vi "Autonomous Independent.vi"() -> ()   [LabVIEW 2011]
doc: "This VI is called when autonomous begins, and will automatically be terminated when autonomous ends. You can carry out timed or sensor driven robot movement independently without needing to return to the caller."
uses:
  <vilib>/Rock Robotics/WPI/Relay/WPI_RelayValue.ctl
  Robot Global Data.vi
  <vilib>/addons/control/pid/pid.llb/PID (DBL).vi
  <vilib>/addons/control/pid/NI_PID_pid.lvlib
  <vilib>/Analysis/NI_AALBase.lvlib
panel:
  out "RPM Control 3":dbl
  out "Target Distance 3":dbl
  out "Turret Stable? 4":bool
  out "State 4":i32
  out "Numeric 4":i32
  in  "Pulse Width (sec) 4":dbl(knob)=0.5086712930755795 scale=0.0..4.0
  out "In Range? 4":bool
  out "RPM Control 2":dbl
  out "Target Distance 2":dbl
  out "Turret Stable? 3":bool
  out "State 3":i32
  out "Numeric 3":i32
  in  "Pulse Width (sec) 3":dbl(knob)=0.5086712930755795 scale=0.0..4.0
  out "In Range? 3":bool
  out "Report":i32
  out "A2: F2":i32
  out "A2: S2":i32
  out "A2: P2":i32
  out "A2: F1":i32
  out "A2: S1":i32
  out "Prime 1":i32
  out "Edge 1":bool
  out "Count 1":bool
  out "Edge 2":bool
  out "count 2":bool
  out "Fire 1":i32
  out "Shooter Stab 1":i32
  out "Fire":i32
  out "Shooter Stable":i32
  out "RPM Control":dbl
  out "Target Distance":dbl
  out "Shooter RPM Response 2":dbl
  out "Waveform Chart 2":cluster{"Shooter RPM Response":dbl, i16}(graph) caption="Waveform Chart"
  out "Turret Stable? 2":bool
  out "State 2":i32
  out "Numeric 2":i32
  in  "Pulse Width (sec) 2":dbl(knob)=0.5086712930755795 scale=0.0..4.0
  out "In Range? 2":bool
  out "In Range?":bool
  in  "Pulse Width (sec)":dbl(knob)=0.5086712930755795 scale=0.0..4.0
  out "Numeric":i32
  out "Turret Stable?":bool
  out "State":i32
  out "Shooter RPM Response":dbl
  in  "Intake Delay (sec)":dbl(knob)=0.15160369527651382 scale=0.0..1.0
  in  "Auto Target Tol (deg)":dbl=1.0
  out "Auton Mode":u32
  in  "Bridge Ball Timeout (sec) 4":dbl=14.5
  out "x-y 61":dbl
  out "x-y 60":dbl
  in  "Prop 4":dbl(knob)=0.059181315414781936 scale=0.0..0.1
  in  "Int 4":dbl(knob) scale=0.0..0.2
  in  "Deriv 4":dbl(knob)=0.030506642412339725 scale=0.0..0.1
  out "RPM Control Response 4":cluster{"setpoint":dbl, "Angle":dbl}(graph)
  out "PID Output 4":dbl(graph)
  out "x-y 56":dbl
  out "x-y 43":dbl
  out "x-y 42":dbl
  in  "Ball 1 Timeout (sec) 5":dbl=6.0
  in  "Prop 2":dbl(knob)=0.059181315414781936 scale=0.0..0.1
  in  "Int 2":dbl(knob) scale=0.0..0.2
  in  "Deriv 2":dbl(knob)=0.030506642412339725 scale=0.0..0.1
  out "RPM Control Response 2":cluster{"setpoint":dbl, "Angle":dbl}(graph)
  out "PID Output 2":dbl(graph)
  out "x-y 34":dbl
  out "x-y 32":dbl
  out "x-y 31":dbl
  in  "Ball 2 Timeout (sec) 4":dbl=8.0
  out "x-y 30":dbl
  out "x-y 29":dbl
  out "x-y 28":dbl
  in  "Ball 1 Timeout (sec) 4":dbl=6.0
  out "x-y 27":dbl
  out "x-y 26":dbl
  in  "Ball 2 Timeout (sec) 3":dbl=12.0
  out "Shooter Ready? 4":bool
  out "x-y 25":dbl
  out "x-y 24":dbl
  out "x-y 23":dbl
  in  "Ball 1 Timeout (sec) 3":dbl=7.0
  out "x-y 22":dbl
  out "x-y 21":dbl
  out "x-y 20":dbl
  in  "Ball 2 Timeout (sec) 2":dbl=12.0
  out "x-y 19":dbl
  out "x-y 18":dbl
  out "x-y 17":dbl
  in  "Ball 1 Timeout (sec) 2":dbl=7.0
  out "x-y 16":dbl
  out "x-y 15":dbl
  in  "Bridge Timeout (sec)":dbl=10.0
  out "x-y 14":dbl
  in  "Bridge Wait Time":dbl=3.0
  out "x-y 7":dbl
  out "x-y 6":dbl
  out "x-y 5":dbl
  out "x-y 4":dbl
  out "x-y 3":dbl
  out "x-y 2":dbl
  out "x-y":dbl
  in  "Ball 1 Timeout (sec)":dbl=6.0
  in  "Ball 2 Timeout (sec)":dbl=8.0
  out "PID Output":dbl(graph)
  in  "Deriv":dbl(knob)=0.030506642412339725 scale=0.0..0.1
  in  "Int":dbl(knob) scale=0.0..0.2
  in  "Prop":dbl(knob)=0.059181315414781936 scale=0.0..0.1
  out "RPM Control Response":cluster{"setpoint":dbl, "Angle":dbl}(graph)
  in  "Drive Brake 'Speed'":dbl=-0.25
  in  "Bridge Actuator Up Time":dbl=0.7
  in  "Bridge Shooter RPM":dbl(knob)=2375.3275564878513 scale=0.0..3000.0
  in  "Bridge Actuator Down Time":dbl=0.7
  in  "Drive Speed":dbl(knob)=0.7003240287631072 scale=0.0..1.0
  in  "Drive Distance (in)":dbl=52.0
  in  "Key Shooter RPM":dbl(knob)=2129.320851431791 scale=0.0..3000.0
  # "0.00228834"
  # "5.2917"
  # "5.86597"
  # "6.97894"
  # "8.73895"
  # "9.44921"
  # "11.5852"
  # "Tol = 25 RPM"
  # "0.00236416"
  # "5.12686"
  # "5.65754"
  # "6.9858"
  # "9.2698"
  # "9.95681"
  # "12.0508"
  # "Fire Ball 1"
  # "Shooter Stable?"
  # "Drive to Bridge"
  # "Wait for Intake"
  # "Shooter at RPM"
  # "Re-Prime for Ball 2"
  # "Fire Ball 2"
  # "Push Bridge"
  # "0.00585747"
  # "3.96963"
  # "4.19854"
  # "4.7273"
  # "6.06736"
  # "6.50122"
  # "7.63292"
  # "8.43019"
  # "14.7075"
  # "0.0028162"
  # "3.90909"
  # "4.35412"
  # "5.11691"
  # "7.55852"
  # "8.06268"
  # "9.35977"
  # "10.1718"
  # "14.7173"
  # "0.0742593"
  # "4.51218"
  # "5.00045"
  # "5.66034"
  # "7.27621"
  # "7.7194"
  # "9.01324"
  # "0"
  # "0"
  # "7.69482"
  # "12.2315"
  # "12.799"
  # "0.00151539"
  # "7.25307"
  # "8.87523"
  # "14.7224"
  # "Tol = 15 RPM"
  # "11.2711"
  # "11.7239"
  # "8.43608"
  # "6.5389"
  # "7.09492"
  # "13.7465"
  # "0.00176096"
  # "Was 0.25 at St.Louis"
  # "Cheas Match 1 was 48\""
  # "48 Inch from curve of Key to Bridge"
  # "Fairgrounds was 2415"
  # "Cheas Practice was 2325"
  # "Cheas Start was 2375"
  # "At RPM"
  # "Fire B1"
  # "Prime B2"
  # "At RPM"
  # "Fire B2"
  # "Auton #2"
  # "0.12688"
  # "10.6952"
  # "11.3261"
  # "12.7335"
  # "13.8453"
  # "14.5186"
types:
  T1 = typedef "WPI_EncoderDevRef.ctl" = cluster{"DevStatus":errorcluster, "EncoderIndex":T2, "CounterIndex":T3, "DistancePerCount":dbl, "Decoding Type":T4}
  T2 = typedef "FPGA_EncoderIdx.ctl" = enum8{"Enc 0", "Enc 1", "Enc 2", "Enc 3", "Invalid"}
  T3 = typedef "FPGA_CounterCtrSystemIndex.ctl" = enum8{"Ctr 0", "Ctr 1", "Ctr 2", "Ctr 3", "Ctr 4", "Ctr 5", "Ctr 6", "Ctr 7", "Invalid"}
  T4 = typedef "WPI_EncoderType.ctl" = enum16{"1x", "2x", "4x"}
  T5 = typedef "WPI_GyroDevRef.ctl" = cluster{"DevStatus":errorcluster, "Analog Module":T6, "Analog Channel":T7, "Offset":dbl, "Gain (VoltsPerDegree/Second)":dbl}
  T6 = typedef "FPGA_TypedefAnalogModule.ctl" = enum16{"Analog Module 1", "Analog Module 2"}
  T7 = typedef "FPGA_AIChannel.ctl" = enum8{"AI 1", "AI 2", "AI 3", "AI 4", "AI 5", "AI 6", "AI 7", "AI 8", "Invalid"}
  T8 = typedef "WPI_DigitalInputDevRef.ctl" = cluster{"DevStatus":errorcluster, "DIO Channel":T9, "Digital Module":T10}
  T9 = typedef "FPGA_DIOChannel.ctl" = enum8{"DIO 1", "DIO 2", "DIO 3", "DIO 4", "DIO 5", "DIO 6", "DIO 7", "DIO 8", "DIO 9", "DIO 10", "DIO 11", "DIO 12", "DIO 13", "DIO 14", "Invalid"}
  T10 = typedef "FPGA_TypedefDigitalModule.ctl" = enum16{"Digital Module 1", "Digital Module 2"}
  T11 = typedef "WPI_RelayDevRef.ctl" = cluster{"DevStatus":errorcluster, "Relay Channel":T12, "Digital Module":T10, "Relay Direction":T13}
  T12 = typedef "FPGA_DIORelayChannel.ctl" = enum8{"Relay 1", "Relay 2", "Relay 3", "Relay 4", "Relay 5", "Relay 6", "Relay 7", "Relay 8", "Invalid"}
  T13 = typedef "WPI_RelayDirection.ctl" = enum16{"Both directions", "Forward only", "Reverse only"}
  T14 = typedef "WPI_RelayValue.ctl" = enum16{"Off", "On", "Forward", "Reverse"}
  T15 = cluster{"Target Distance":dbl, "Target Distance":dbl, "Target Distance":dbl, "Target Distance":dbl, "Target Distance":dbl}
  T16 = cluster{"Prop 2":dbl, "Int 2":dbl, "Deriv 2":dbl}
  T17 = cluster{"Prop 4":dbl, "Int 4":dbl, "Deriv 4":dbl}
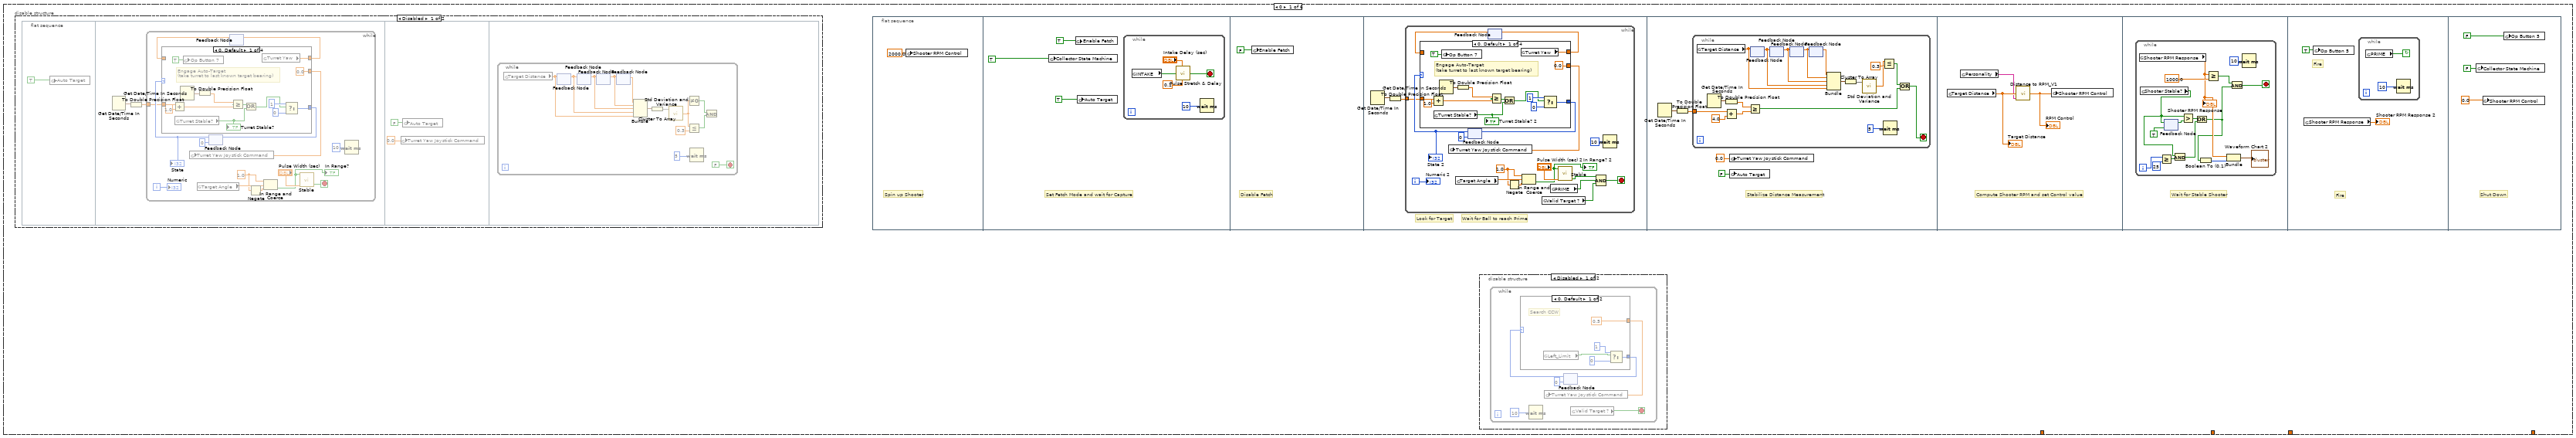
[diagram p2: hidden frame]
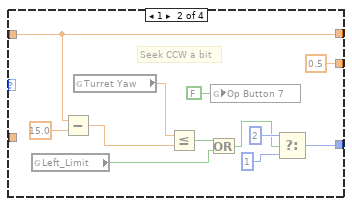
[diagram p3: hidden frame]
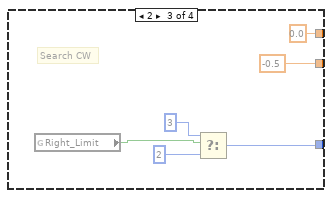
[diagram p4: hidden frame]
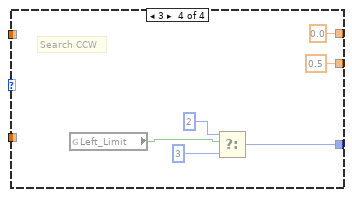
[diagram p5: hidden frame]
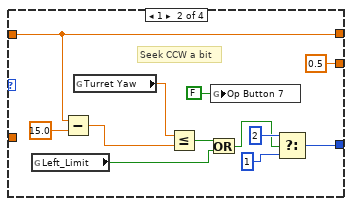
[diagram p7: hidden frame]
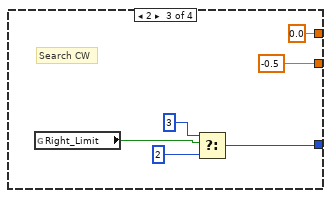
[diagram p8: hidden frame]
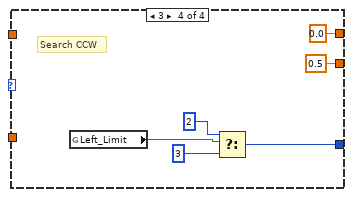
[diagram p9: hidden frame]
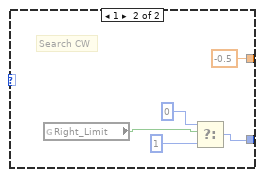
[diagram p10: hidden frame]
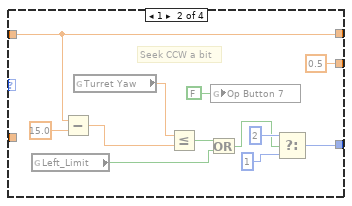
[diagram p16: hidden frame]
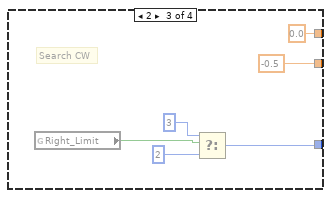
[diagram p17: hidden frame]
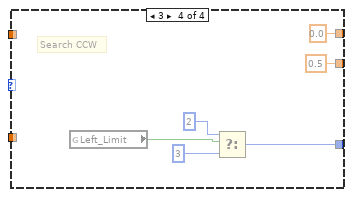
[diagram p18: hidden frame]
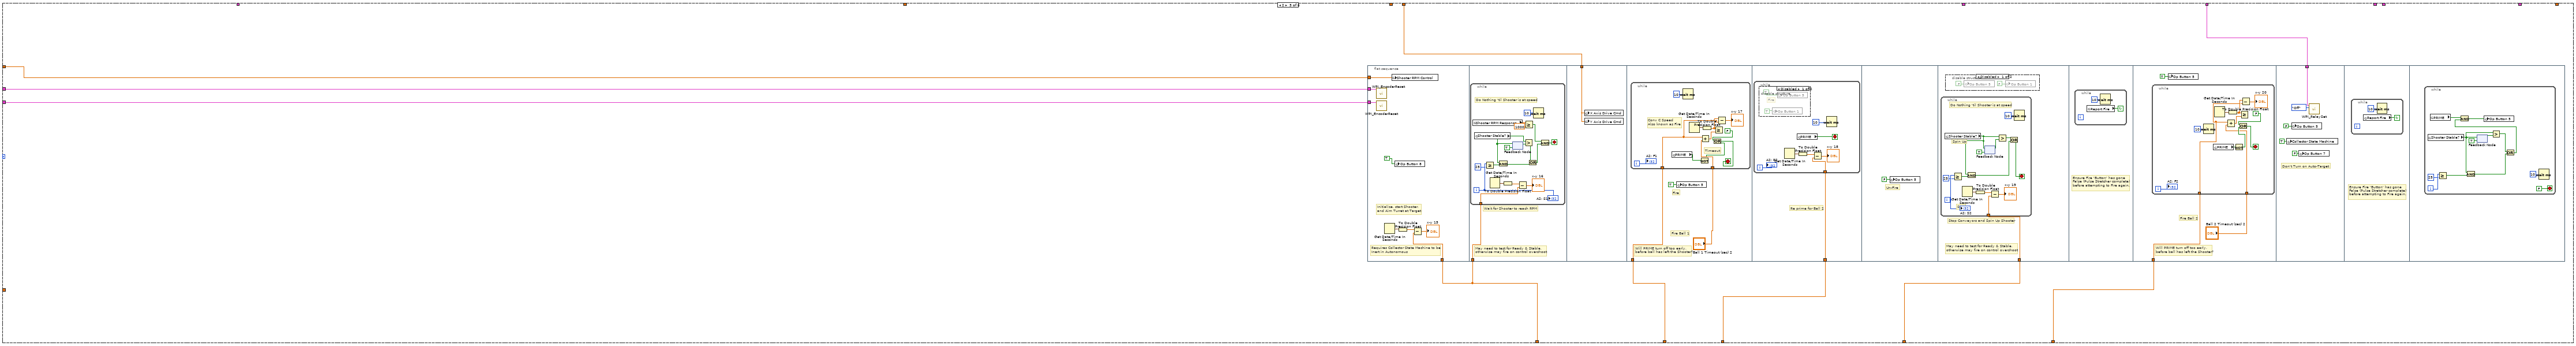
[diagram p19: hidden frame]
diagram:
  (unwired) "This code sets the toggle rate used by the Periodic Tasks VI.  For autonomous mode we slowly flash the USER1 LED on the cRIO.  Look at the Periodic Tasks VI to see how this global value is used."
  (unwired) "This function is run in parallel when the autonomous period begins. It will be terminated automatically when the period ends.\n\nNote that all Driver Station inputs are automatically latched and will not change once auto begins."
  # "Initial condition is Robot Turret is aimed at Target.\nUse this to create the initial Target Bearing."
  # "The different autonomous can be set up from\nthe driver station. Set up as binary.\n\n1 (001) - Default\n\n2 (010)- Coopertition (have another bot feed us balls \nthat we can shoot, NO BRIDGE)\n\n3 (011)- X second delay to shooting first ball (NO BRIDGE)\n\n4 (100) - X second delay to shooting first ball (Go for bridge)\n\n5 (101)- Reverse Order (Puts down bridge then shoots)"
  # "Every 20ms, report that we are running autonomous\ncode. Loop will abort the same time as the VI."
  # "This tells you the driver position\nand alliance color"
  # "This gives you the eight Driver Station\ndigital switch settings"
  # "This gives you the four\nDriver Station sliders or\nanalog voltages"
  n1 = global read "Robot Global Data.vi" "Turret Yaw"() -> (w5:dbl)
  n2 = global read "Robot Global Data.vi" "Robot Gyro"() -> (w4:dbl)
  n3 = global write "Robot Global Data.vi" "Collector State Machine"(TRUE ("Collector State Machine")) -> ()
  n4 = global write "Robot Global Data.vi" "Autonomous Drive"(TRUE ("Autonomous Drive")) -> ()
  n5 = global write "Robot Global Data.vi" "Shooter RPM Tol"(25.0 ("Shooter RPM Tol")) -> ()
  n6 = global write "Robot Global Data.vi" "Op Button 9"(FALSE ("Op Button 9")) -> ()
  n7 = global write "Robot Global Data.vi" "Op Button 5"(FALSE ("Op Button 9")) -> ()
  n8 = global write "Robot Global Data.vi" "Op Button 7"(FALSE ("Dr Button 5")) -> ()
  n9 = global write "Robot Global Data.vi" "Auto Target"(FALSE ("Auto Target")) -> ()
  n10 = Add(x=w5, y=w4) -> (x+y=w3:dbl)
  n11 = call "Gyro Angle.vi"("Mod"=360.0, "Input"=w3) -> ("Output"=w2:dbl)  [unwired: 9 in]
  n12 = global write "Robot Global Data.vi" "Target Bearing"(w2) -> ()
  n13 = call <vilib>:"WPI_DriverStationGet Digital Input.vi"() -> ("Driver Station Digital Input (1-8)"=w16:bool[])  [unwired: 11 in]
  n14 = Index Array(array=w16, index=3) -> (element=w12:bool)
  n15 = Index Array(array=w16, index=2) -> (element=w15:bool)
  n16 = Index Array(array=w16, index=1) -> (element=w11:bool)
  n17 = call <vilib>:"WPI_EncoderRefNum Registry Get.vi"("refnum name"="Right Wheel Encoder") -> ("EncoderDevRef"=w38:T1)  [unwired: 9 in, 1 out]
  n18 = call <vilib>:"WPI_EncoderRefNum Registry Get.vi"("refnum name"="Left Wheel Encoder") -> ("EncoderDevRef"=w39:T1)  [unwired: 9 in, 1 out]
  n19 = Bundle(w12, w15, w11) -> (w14:cluster{bool, bool, bool})  [unwired: 1 in]
  n20 = call <vilib>:"WPI_DriverStationGet Analog Input.vi"() -> ("Analog 1 (V)"=w29:dbl)  [unwired: 8 in, 3 out]
  n21 = Cluster To Array(cluster=w14) -> (array=w13:bool[])
  n22 = Boolean Array To Number(Boolean array=w13) -> (number=w30:u32)
  "Auton Mode" <- w30
  n23 = call <vilib>:"WPI_DriverStationSet Digital Output.vi"("Driver Station Digital Output (1-8)"=w13) -> ()  [unwired: 10 in, 1 out]
  n24 = Get Date/Time In Seconds() -> (seconds since 1Jan1904=w10:timestamp)
  n25 = To Double Precision Float(number=w10) -> (double precision float=w9:dbl)
  n26 = while {
    stop <- FALSE stop-if-true
    n27 = call <vilib>:"WPI_DriverStationReport Robot Code State.vi"("Autonomous"=TRUE) -> ()  [unwired: 10 in, 1 out]
    n28 = Wait (ms)(milliseconds to wait=u32 20) -> ()  [unwired: 1 out]
  }
  n29 = call <vilib>:"WPI_DriverStationGet Alliance Info.vi"() -> ()  [unwired: 12 out]
  n30 = call <vilib>:"WPI_DriverStationGet Digital Input.vi"() -> ("Driver Station Digital Input (1-8)"=w46:bool[])  [unwired: 11 out]
  n31 = call <vilib>:"WPI_DriverStationGet Analog Input.vi"() -> ()  [unwired: 12 out]
  n32 = Index Array(array=w46) -> ()  [unwired: 8 in, 8 out]
  n33 = global write "Robot Global Data.vi" "LED toggle rate (ms)"(u32 500 ("LED ms toggle rate")) -> ()
  n34 = call <vilib>:"WPI_GyroRefNum Registry Get.vi"("refnum name"="Robot Gyro") -> ("GyroDevRef"=w26:T5)  [unwired: 9 in, 1 out]
  n35 = call <vilib>:"WPI_DigitalInputRefNum Registry Get.vi"("refnum name"="Bridge Actuator Down") -> ("DigitalInputDevRef"=w31:T8)  [unwired: 9 in, 1 out]
  n36 = call <vilib>:"WPI_RelayRefNum Registry Get.vi"("refnum name"="Bridge Actuator") -> ("RelayDevRef"=w27:T11)  [unwired: 9 in, 1 out]
  n37 = case shown="1, Default" w30 {
    tunnel: "Drive Speed" -> [_ w264 _ _ w761 w919]
    tunnel: "Drive Distance (in)" -> [_ w263 _ _ w760 w918]
    tunnel: "Key Shooter RPM" -> [_ w262 w510 w636 w758 _]
    tunnel: w39 -> [_ w261 w519 w638 w757 w924]
    tunnel: w38 -> [_ w260 w518 w637 w756 w925]
    tunnel: "Bridge Actuator Down Time" -> [_ _ _ _ _ _]
    tunnel: "Bridge Shooter RPM" -> [_ w259 _ _ w763 w914]
    tunnel: "Drive Brake 'Speed'" -> [_ w258 w517 w635 w755 _]
    tunnel: w26 -> [_ w257 _ _ w762 _]
    tunnel: "Bridge Actuator Up Time" -> [_ _ _ _ _ _]
    tunnel: "Bridge Wait Time" -> [_ _ _ _ _ _]
    tunnel: w9 -> [_ w256 w514 w632 w753 w916]
    tunnel: w31 -> [_ w255 _ _ _ w922]
    tunnel: w27 -> [_ w254 _ _ _ _]
    tunnel: w9 -> [_ _ w516 w630 w754 w917]
    tunnel: w9 -> [_ _ w515 w633 _ _]
    tunnel: w9 -> [_ _ w513 w629 w752 _]
    tunnel: w9 -> [_ _ w512 _ w750 w915]
    tunnel: w27 -> [_ _ w511 _ _ _]
    tunnel: w29 -> [_ _ _ w634 w749 _]
    tunnel: w26 -> [_ _ _ _ w759 _]
    tunnel: w27 -> [_ _ _ _ _ w921]
    tunnel: "Drive Brake 'Speed'" -> [_ _ _ _ w751 _]
    tunnel: "Bridge Actuator Up Time" -> [_ _ _ _ _ _]
    tunnel: w27 -> [_ _ _ w631 _ _]
    tunnel: "Drive Brake 'Speed'" -> [_ _ _ _ _ w923]
    tunnel: w26 -> [_ _ _ _ _ _]
    tunnel: w26 -> [_ _ _ _ _ w920]
    tunnel: "Drive Brake 'Speed'" -> [_ _ _ _ _ w913]
    tunnel: "Auto Target Tol (deg)" -> [_ w253 _ _ w748 w910]
    tunnel: "Auto Target Tol (deg)" -> [_ _ _ _ _ w909]
    frame 0 {
      n38 = disable-structure shown="Disabled" {
        frame Disabled {
          n39 = flat-sequence {
            frame #0 {
              n40 = global write "Robot Global Data.vi" "Auto Target"(TRUE ("Auto Target")) -> ()
            }
            frame #1 {
              n41 = Get Date/Time In Seconds() -> (seconds since 1Jan1904=w52:timestamp)
              n42 = To Double Precision Float(number=w52) -> (double precision float=w51:dbl)
              n43 = while {
                tunnel: w51 -> [w62]
                i -> [w61]
                stop <- w55 stop-if-true
                w56 = 1.0 ("upper limit")
                n44 = global read "Robot Global Data.vi" "Target Angle"() -> (w58:dbl)
                n45 = feedback #1(0) -> (w66:i32)
                "State" <- w66
                n46 = feedback #2() -> (w63:dbl)  [unwired: 1 in]
                n47 = case shown="0, Default" w66 {
                  tunnel: [w79 w90 w97 w104] -> w59
                  tunnel: [0.0 0.5 -0.5 0.5] -> w65
                  tunnel: [w76 w92 0.0 ("Turret Yaw") 0.0 ("Turret Yaw")] -> w64
                  tunnel: w63 -> [_ w92 _ _]
                  tunnel: w62 -> [w71 _ _ _]
                  frame 0, Default {
                    # "Engage Auto-Target\n(take turret to last known target bearing)"
                    n48 = Add(x=w71, y=1.0) -> (x+y=w68:dbl)
                    n49 = global read "Robot Global Data.vi" "Turret Stable?"() -> (w74:bool)
                    "Turret Stable?" <- w74
                    n50 = Get Date/Time In Seconds() -> (seconds since 1Jan1904=w73:timestamp)
                    n51 = global write "Robot Global Data.vi" "Op Button 7"(TRUE ("Op Button 7")) -> ()
                    n52 = To Double Precision Float(number=w73) -> (double precision float=w69:dbl)
                    n53 = Greater Or Equal?(x=w69, y=w68) -> (x >= y?=w72:bool)
                    n54 = Or(x=w72, y=w74) -> (x .or. y?=w75:bool)
                    n55 = global read "Robot Global Data.vi" "Turret Yaw"() -> (w76:dbl)
                    n56 = Select(t=1, s=w75, f=0) -> (s? t:f=w79:i32)
                  }
                  frame 1 {
                    # "Seek CCW a bit"
                    n57 = global read "Robot Global Data.vi" "Left_Limit"() -> (w82:bool)
                    n58 = Subtract(x=w92, y=15.0) -> (x-y=w86:dbl)
                    n59 = global read "Robot Global Data.vi" "Turret Yaw"() -> (w87:dbl)
                    n60 = Less Or Equal?(x=w87, y=w86) -> (x <= y?=w84:bool)
                    n61 = Or(x=w84, y=w82) -> (x .or. y?=w83:bool)
                    n62 = global write "Robot Global Data.vi" "Op Button 7"(FALSE ("Op Button 7")) -> ()
                    n63 = Select(t=2, s=w83, f=1) -> (s? t:f=w90:i32)
                  }
                  frame 2 {
                    # "Search CW"
                    n64 = global read "Robot Global Data.vi" "Right_Limit"() -> (w94:bool)
                    n65 = Select(t=3, s=w94, f=2) -> (s? t:f=w97:i32)
                  }
                  frame 3 {
                    # "Search CCW"
                    n66 = global read "Robot Global Data.vi" "Left_Limit"() -> (w100:bool)
                    n67 = Select(t=2, s=w100, f=3) -> (s? t:f=w104:i32)
                  }
                }
                n68 = global write "Robot Global Data.vi" "Turret Yaw Joystick Command"(w65) -> ()
                n69 = feedback-in #1(w59) -> ()
                n70 = feedback-in #2(w64) -> ()
                n71 = Negate(x=w56) -> (-x=w57:dbl)
                n72 = In Range and Coerce(upper limit=w56, x=w58, lower limit=w57) -> (In Range?=w54:bool)  [unwired: 1 out]
                "In Range?" <- w54
                n73 = call "Stable.vi"("Pulse Width (sec)"="Pulse Width (sec)", "Signal Input"=w54) -> ("Stable"=w55:bool)  [unwired: 9 in]
                n74 = Wait (ms)(milliseconds to wait=u32 10) -> ()  [unwired: 1 out]
                "Numeric" <- w61
              }
            }
            frame #2 {
              n75 = global write "Robot Global Data.vi" "Turret Yaw Joystick Command"(0.0 ("Turret Yaw Joystick Command")) -> ()
              n76 = global write "Robot Global Data.vi" "Auto Target"(FALSE ("Auto Target")) -> ()
            }
            frame #3 {
              n77 = while {
                stop <- FALSE stop-if-true
                n78 = global read "Robot Global Data.vi" "Target Distance"() -> (w109:dbl)
                n79 = feedback #3() -> (w117:dbl)  [unwired: 1 in]
                n80 = feedback-in #3(w109) -> ()
                n81 = feedback #4() -> (w118:dbl)  [unwired: 1 in]
                n82 = feedback-in #4(w117) -> ()
                n83 = feedback #5() -> (w119:dbl)  [unwired: 1 in]
                n84 = feedback-in #5(w118) -> ()
                n85 = feedback #6() -> (w120:dbl)  [unwired: 1 in]
                n86 = feedback-in #6(w119) -> ()
                n87 = Bundle("Target Distance"=w120, "Target Distance"=w119, "Target Distance"=w118, "Target Distance"=w117, "Target Distance"=w109) -> (w116:T15)  [unwired: 1 in]
                n88 = Cluster To Array(cluster=w116) -> (array=w115:dbl[])
                n89 = call <vilib>:"Std Deviation and Variance.vi"("X"=w115) -> ("standard deviation"=w108:dbl)  [unwired: 1 in, 2 out]
                n90 = Not Equal To 0?(x=w108) -> (x != 0?=w113:bool)
                n91 = Less Or Equal?(x=w108, y=0.3) -> (x <= y?=w112:bool)
                n92 = Wait (ms)(milliseconds to wait=u32 5) -> ()  [unwired: 1 out]
                n93 = And(x=w113, y=w112) -> ()  [unwired: 1 out]
              }
            }
          }
        }
        frame Enabled {
        }
      }
      n94 = flat-sequence {
        frame #0 {
          # "Spin up Shooter"
          n95 = global write "Robot Global Data.vi" "Shooter RPM Control"(2000.0 ("Shooter RPM Control")) -> ()
        }
        frame #1 {
          # "Set Fetch Mode and wait for Capture"
          n96 = global write "Robot Global Data.vi" "Collector State Machine"(TRUE ("Collector State Machine")) -> ()
          n97 = global write "Robot Global Data.vi" "Enable Fetch"(TRUE ("Enable Fetch")) -> ()
          n98 = global write "Robot Global Data.vi" "Auto Target"(TRUE ("Auto Target")) -> ()
          n99 = while {
            stop <- w126 stop-if-true
            n100 = global read "Robot Global Data.vi" "INTAKE"() -> (w125:bool)
            n101 = call "Pulse Stretch & Delay.vi"("Delay (sec)"="Intake Delay (sec)", "In"=w125, "Width (sec)"=0.1) -> ("Out"=w126:bool)  [unwired: 2 in]
            n102 = Wait (ms)(milliseconds to wait=u32 10) -> ()  [unwired: 1 out]
          }
        }
        frame #2 {
          # "Disable Fetch"
          n103 = global write "Robot Global Data.vi" "Enable Fetch"(FALSE ("Enable Fetch")) -> ()
        }
        frame #3 {
          # "Wait for Ball to reach Prime"
          # "Look for Target"
          n104 = Get Date/Time In Seconds() -> (seconds since 1Jan1904=w131:timestamp)
          n105 = To Double Precision Float(number=w131) -> (double precision float=w132:dbl)
          n106 = while {
            tunnel: w132 -> [w145]
            i -> [w144]
            stop <- w134 stop-if-true
            w139 = 1.0 ("upper limit")
            n107 = global read "Robot Global Data.vi" "Target Angle"() -> (w141:dbl)
            n108 = feedback #7(0) -> (w149:i32)
            "State 2" <- w149
            n109 = feedback #8() -> (w146:dbl)  [unwired: 1 in]
            n110 = case shown="0, Default" w149 {
              tunnel: [w162 w173 w180 w187] -> w142
              tunnel: [0.0 0.5 -0.5 0.5] -> w148
              tunnel: [w159 w175 0.0 ("Turret Yaw") 0.0 ("Turret Yaw")] -> w147
              tunnel: w146 -> [_ w175 _ _]
              tunnel: w145 -> [w154 _ _ _]
              frame 0, Default {
                # "Engage Auto-Target\n(take turret to last known target bearing)"
                n111 = Add(x=w154, y=1.0) -> (x+y=w151:dbl)
                n112 = global read "Robot Global Data.vi" "Turret Stable?"() -> (w157:bool)
                "Turret Stable? 2" <- w157
                n113 = Get Date/Time In Seconds() -> (seconds since 1Jan1904=w156:timestamp)
                n114 = global write "Robot Global Data.vi" "Op Button 7"(TRUE ("Op Button 7")) -> ()
                n115 = To Double Precision Float(number=w156) -> (double precision float=w152:dbl)
                n116 = Greater Or Equal?(x=w152, y=w151) -> (x >= y?=w155:bool)
                n117 = Or(x=w155, y=w157) -> (x .or. y?=w158:bool)
                n118 = global read "Robot Global Data.vi" "Turret Yaw"() -> (w159:dbl)
                n119 = Select(t=1, s=w158, f=0) -> (s? t:f=w162:i32)
              }
              frame 1 {
                # "Seek CCW a bit"
                n120 = global read "Robot Global Data.vi" "Left_Limit"() -> (w165:bool)
                n121 = Subtract(x=w175, y=15.0) -> (x-y=w169:dbl)
                n122 = global read "Robot Global Data.vi" "Turret Yaw"() -> (w170:dbl)
                n123 = Less Or Equal?(x=w170, y=w169) -> (x <= y?=w167:bool)
                n124 = Or(x=w167, y=w165) -> (x .or. y?=w166:bool)
                n125 = global write "Robot Global Data.vi" "Op Button 7"(FALSE ("Op Button 7")) -> ()
                n126 = Select(t=2, s=w166, f=1) -> (s? t:f=w173:i32)
              }
              frame 2 {
                # "Search CW"
                n127 = global read "Robot Global Data.vi" "Right_Limit"() -> (w177:bool)
                n128 = Select(t=3, s=w177, f=2) -> (s? t:f=w180:i32)
              }
              frame 3 {
                # "Search CCW"
                n129 = global read "Robot Global Data.vi" "Left_Limit"() -> (w183:bool)
                n130 = Select(t=2, s=w183, f=3) -> (s? t:f=w187:i32)
              }
            }
            n131 = global write "Robot Global Data.vi" "Turret Yaw Joystick Command"(w148) -> ()
            n132 = feedback-in #7(w142) -> ()
            n133 = feedback-in #8(w147) -> ()
            n134 = Negate(x=w139) -> (-x=w140:dbl)
            n135 = In Range and Coerce(upper limit=w139, x=w141, lower limit=w140) -> (In Range?=w138:bool)  [unwired: 1 out]
            "In Range? 2" <- w138
            n136 = global read "Robot Global Data.vi" "Valid Target ?"() -> (w133:bool)
            n137 = global read "Robot Global Data.vi" "PRIME"() -> (w135:bool)
            n138 = call "Stable.vi"("Pulse Width (sec)"="Pulse Width (sec) 2", "Signal Input"=w138) -> ("Stable"=w136:bool)  [unwired: 9 in]
            n139 = Compound Arithmetic op=AND(w136, w135, w133) -> (w134:bool)
            n140 = Wait (ms)(milliseconds to wait=u32 10) -> ()  [unwired: 1 out]
            "Numeric 2" <- w144
          }
        }
        frame #4 {
          # "Stabilize Distance Measurement"
          n141 = Get Date/Time In Seconds() -> (seconds since 1Jan1904=w190:timestamp)
          n142 = To Double Precision Float(number=w190) -> (double precision float=w189:dbl)
          n143 = while {
            tunnel: w189 -> [w197]
            stop <- w200 stop-if-true
            n144 = global read "Robot Global Data.vi" "Target Distance"() -> (w202:dbl)
            n145 = Get Date/Time In Seconds() -> (seconds since 1Jan1904=w199:timestamp)
            n146 = To Double Precision Float(number=w199) -> (double precision float=w196:dbl)
            n147 = Add(x=w197, y=4.0) -> (x+y=w195:dbl)
            n148 = Greater Or Equal?(x=w196, y=w195) -> (x >= y?=w193:bool)
            n149 = feedback #9() -> (w207:dbl)  [unwired: 1 in]
            n150 = feedback-in #9(w202) -> ()
            n151 = feedback #10() -> (w208:dbl)  [unwired: 1 in]
            n152 = feedback-in #10(w207) -> ()
            n153 = feedback #11() -> (w209:dbl)  [unwired: 1 in]
            n154 = feedback-in #11(w208) -> ()
            n155 = feedback #12() -> (w210:dbl)  [unwired: 1 in]
            n156 = feedback-in #12(w209) -> ()
            n157 = Bundle("Target Distance"=w210, "Target Distance"=w209, "Target Distance"=w208, "Target Distance"=w207, "Target Distance"=w202) -> (w206:T15)  [unwired: 1 in]
            n158 = Cluster To Array(cluster=w206) -> (array=w205:dbl[])
            n159 = call <vilib>:"Std Deviation and Variance.vi"("X"=w205) -> ("standard deviation"=w201:dbl)  [unwired: 1 in, 2 out]
            n160 = Less Or Equal?(x=w201, y=0.3) -> (x <= y?=w194:bool)
            n161 = Wait (ms)(milliseconds to wait=u32 5) -> ()  [unwired: 1 out]
            n162 = Or(x=w194, y=w193) -> (x .or. y?=w200:bool)
          }
          n163 = global write "Robot Global Data.vi" "Turret Yaw Joystick Command"(0.0 ("Turret Yaw Joystick Command")) -> ()
          n164 = global write "Robot Global Data.vi" "Auto Target"(FALSE ("Auto Target")) -> ()
        }
        frame #5 {
          # "Compute Shooter RPM and set Control value"
          n165 = global read "Robot Global Data.vi" "Target Distance"() -> (w212:dbl)
          "Target Distance" <- w212
          n166 = global read "Robot Global Data.vi" "Personality"() -> (w211:string)
          n167 = call "Distance to RPM_V1.vi"("Personality"=w211, "Target Distance"=w212) -> ("Shooter RPM Control"=w213:dbl)  [unwired: 3 in]
          "RPM Control" <- w213
          n168 = global write "Robot Global Data.vi" "Shooter RPM Control"(w213) -> ()
        }
        frame #6 {
          # "Wait for Stable Shooter"
          n169 = while {
            i -> [w218]
            stop <- w223 stop-if-true
            n170 = global read "Robot Global Data.vi" "Shooter RPM Response"() -> (w226:dbl)
            "Shooter RPM Response" <- w226
            n171 = global read "Robot Global Data.vi" "Shooter Stable?"() -> (w215:bool)
            n172 = Greater Or Equal?(x=w218, y=25) -> (x >= y?=w216:bool)
            n173 = feedback #13(TRUE ("Shooter Stable?")) -> (w221:bool)
            n174 = feedback-in #13(w215) -> ()
            n175 = And(x=w215, y=w216) -> (x .and. y?=w214:bool)
            n176 = Greater?(x=w215, y=w221) -> (0:w220:bool)
            n177 = Or(x=w220, y=w214) -> (x .or. y?=w219:bool)
            n178 = Boolean To (0,1)(Boolean=w219) -> (0, 1=w225:i16)
            n179 = Greater Or Equal?(x=w226, y=1000.0) -> (x >= y?=w227:bool)
            n180 = Bundle("Shooter RPM Response"=w226, w225) -> (→"Waveform Chart 2":cluster{"Shooter RPM Response":dbl, i16})  [unwired: 1 in]
            n181 = And(x=w227, y=w219) -> (x .and. y?=w223:bool)
            n182 = Wait (ms)(milliseconds to wait=u32 10) -> ()  [unwired: 1 out]
          }
        }
        frame #7 {
          # "Fire"
          # "Fire"
          n183 = global read "Robot Global Data.vi" "Shooter RPM Response"() -> (→"Shooter RPM Response 2":dbl)
          n184 = global write "Robot Global Data.vi" "Op Button 5"(TRUE ("Op Button 5")) -> ()
          n185 = while {
            stop <- w233 continue-if-true
            n186 = global read "Robot Global Data.vi" "PRIME"() -> (w233:bool)
            n187 = Wait (ms)(milliseconds to wait=u32 10) -> ()  [unwired: 1 out]
          }
        }
        frame #8 {
          # "Shut Down"
          n188 = global write "Robot Global Data.vi" "Collector State Machine"(FALSE ("Collector State Machine")) -> ()
          n189 = global write "Robot Global Data.vi" "Shooter RPM Control"(0.0 ("Shooter RPM Control")) -> ()
          n190 = global write "Robot Global Data.vi" "Op Button 5"(FALSE ("Op Button 5")) -> ()
        }
      }
      n191 = disable-structure shown="Disabled" {
        frame Disabled {
          n192 = while {
            stop <- w242 stop-if-true
            n193 = Wait (ms)(milliseconds to wait=u32 10) -> ()  [unwired: 1 out]
            n194 = feedback #14(0) -> (w238:i32)
            n195 = case shown="0, Default" w238 {
              tunnel: [w246 w249] -> w240
              tunnel: [0.5 ("Turret Yaw Joystick Command") -0.5 ("Turret Yaw Joystick Command")] -> w237
              frame 0, Default {
                # "Search CCW"
                n196 = global read "Robot Global Data.vi" "Left_Limit"() -> (w245:bool)
                n197 = Select(t=1, s=w245, f=0) -> (s? t:f=w246:i32)
              }
              frame 1 {
                # "Search CW"
                n198 = global read "Robot Global Data.vi" "Right_Limit"() -> (w251:bool)
                n199 = Select(t=0, s=w251, f=1) -> (s? t:f=w249:i32)
              }
            }
            n200 = global write "Robot Global Data.vi" "Turret Yaw Joystick Command"(w237) -> ()
            n201 = feedback-in #14(w240) -> ()
            n202 = global read "Robot Global Data.vi" "Valid Target ?"() -> (w242:bool)
          }
        }
        frame Enabled {
        }
      }
    }
    frame 1, Default {
      n203 = flat-sequence {
        tunnel: w262 -> [w272]
        tunnel: w256 -> [w267]
        tunnel: w260 -> [w270]
        tunnel: w261 -> [w271]
        tunnel: w256 -> [w274]
        tunnel: w258 -> [w299]
        tunnel: w256 -> [w302]
        tunnel: w256 -> [w311]
        tunnel: w256 -> [w324]
        tunnel: w256 -> [w349]
        tunnel: w256 -> [w359]
        tunnel: w255 -> [w358]
        tunnel: w254 -> [w357]
        tunnel: w257 -> [w380]
        tunnel: w256 -> [w381]
        tunnel: w257 -> [w382]
        tunnel: w259 -> [w383]
        tunnel: w263 -> [w384]
        tunnel: w264 -> [w385]
        tunnel: w258 -> [w409]
        tunnel: w253 -> [w500]
        frame #0 {
          # "Requires Collector State Machine to be\nInert in Autonomous"
          # "Initialize, start Shooter"
          n204 = call <vilib>:"WPI_EncoderReset.vi"("EncoderDevRef"=w271) -> ()  [unwired: 9 in, 2 out]
          n205 = call <vilib>:"WPI_EncoderReset.vi"("EncoderDevRef"=w270) -> ()  [unwired: 9 in, 2 out]
          n206 = Get Date/Time In Seconds() -> (seconds since 1Jan1904=w269:timestamp)
          n207 = To Double Precision Float(number=w269) -> (double precision float=w268:dbl)
          n208 = global write "Robot Global Data.vi" "Dr Button 2"(TRUE ("Dr Button 5")) -> ()
          n209 = Subtract(x=w268, y=w267) -> (x-y=→"x-y":dbl)
          n210 = global write "Robot Global Data.vi" "Shooter RPM Control"(w272) -> ()
        }
        frame #1 {
          # "May need to test for Ready & Stable,\notherwise may fire on control overshoot"
          # "Wait for Shooter to reach RPM"
          n211 = while {
            tunnel: w274 -> [w285]
            tunnel: "Ball 1 Timeout (sec)" -> [w286]
            i -> [w279]
            stop <- w291 stop-if-true
            # "Timeout"
            # "Do Nothing 'til Shooter is at speed"
            n212 = global read "Robot Global Data.vi" "Shooter RPM Response"() -> (w297:dbl)
            n213 = global read "Robot Global Data.vi" "Shooter Stable?"() -> (w277:bool)
            n214 = Greater Or Equal?(x=w279, y=25) -> (x >= y?=w281:bool)
            n215 = And(x=w277, y=w281) -> (x .and. y?=w278:bool)
            "Count 1" <- w278
            n216 = feedback #15(TRUE ("Shooter Stable?")) -> (w283:bool)
            n217 = feedback-in #15(w277) -> ()
            n218 = Greater Or Equal?(x=w297, y=1000.0) -> (x >= y?=w295:bool)
            n219 = Greater?(x=w277, y=w283) -> (0:w276:bool)
            "Edge 1" <- w276
            n220 = Wait (ms)(milliseconds to wait=u32 10) -> ()  [unwired: 1 out]
            n221 = Or(x=w276, y=w278) -> (x .or. y?=w275:bool)
            n222 = And(x=w295, y=w275) -> (x .and. y?=w287:bool)
            n223 = Get Date/Time In Seconds() -> (seconds since 1Jan1904=w292:timestamp)
            n224 = Or(x=FALSE, y=w287) -> (x .or. y?=w291:bool)
            n225 = To Double Precision Float(number=w292) -> (double precision float=w293:dbl)
            n226 = Get Date/Time In Seconds() -> (seconds since 1Jan1904=w289:timestamp)
            n227 = Subtract(x=w293, y=w285) -> (x-y=→"x-y 2":dbl)
            n228 = Add(x=w285, y=w286) -> (x+y=w288:dbl)
            n229 = To Double Precision Float(number=w289) -> (double precision float=w290:dbl)
            n230 = Greater Or Equal?(x=w290, y=w288) -> ()  [unwired: 1 out]
            "Shooter Stab 1" <- w279
          }
        }
        frame #2 {
          n231 = global write "Robot Global Data.vi" "X Axis Drive Cmd"(w299) -> ()
          n232 = global write "Robot Global Data.vi" "Y Axis Drive Cmd"(w299) -> ()
          n233 = global write "Robot Global Data.vi" "Dr Button 2"(FALSE) -> ()
        }
        frame #3 {
          # "Fire"
          # "Will PRIME turn off too early, \nbefore ball has left the Shooter?"
          # "Fire Ball 1"
          n234 = while {
            tunnel: w302 -> [w306]
            i -> [w303]
            stop <- w304 continue-if-true
            n235 = global read "Robot Global Data.vi" "PRIME"() -> (w304:bool)
            n236 = Get Date/Time In Seconds() -> (seconds since 1Jan1904=w308:timestamp)
            n237 = To Double Precision Float(number=w308) -> (double precision float=w307:dbl)
            n238 = Subtract(x=w307, y=w306) -> (x-y=→"x-y 3":dbl)
            n239 = Wait (ms)(milliseconds to wait=u32 10) -> ()  [unwired: 1 out]
            "Fire 1" <- w303
          }
          n240 = global write "Robot Global Data.vi" "Op Button 5"(TRUE ("Op Button 5")) -> ()
        }
        frame #4 {
          # "Fire Conv Off"
          # "Re prime for Ball 2"
          n241 = while {
            tunnel: w311 -> [w315]
            i -> [w314]
            stop <- w319 stop-if-true
            n242 = Get Date/Time In Seconds() -> (seconds since 1Jan1904=w318:timestamp)
            n243 = To Double Precision Float(number=w318) -> (double precision float=w317:dbl)
            n244 = global read "Robot Global Data.vi" "PRIME"() -> (w319:bool)
            n245 = Subtract(x=w317, y=w315) -> (x-y=→"x-y 4":dbl)
            n246 = Wait (ms)(milliseconds to wait=u32 10) -> ()  [unwired: 1 out]
            "Prime 1" <- w314
          }
          n247 = disable-structure shown="Disabled" {
            frame Disabled {
              # "Fire Conv On"
              # "Mid Conv Forward"
              n248 = global write "Robot Global Data.vi" "Op Button 5"(TRUE ("Op Button 5")) -> ()
              n249 = global write "Robot Global Data.vi" "Op Button 1"(TRUE ("Op Button 5")) -> ()
            }
            frame Enabled {
            }
          }
          n250 = global write "Robot Global Data.vi" "Op Button 5"(FALSE ("Op Button 5")) -> ()
        }
        frame #5 {
          n251 = disable-structure shown="Disabled" {
            frame Disabled {
              # "Mid Conv Off"
              # "Fire Conv Off"
              n252 = global write "Robot Global Data.vi" "Op Button 5"(FALSE ("Op Button 5")) -> ()
              n253 = global write "Robot Global Data.vi" "Op Button 1"(FALSE ("Op Button 5")) -> ()
            }
            frame Enabled {
            }
          }
        }
        frame #6 {
          # "May need to test for Ready & Stable,\notherwise may fire on control overshoot"
          # "Stop Conveyors and Spin Up Shooter"
          # "Spin Up"
          # "Stop"
          n254 = while {
            tunnel: w324 -> [w336]
            tunnel: "Ball 2 Timeout (sec)" -> [w335]
            i -> [w330]
            stop <- w337 stop-if-true
            # "Timeout"
            # "Do Nothing 'til Shooter is at speed"
            n255 = Wait (ms)(milliseconds to wait=u32 10) -> ()  [unwired: 1 out]
            n256 = Greater Or Equal?(x=w330, y=25) -> (x >= y?=w331:bool)
            n257 = Get Date/Time In Seconds() -> (seconds since 1Jan1904=w341:timestamp)
            n258 = To Double Precision Float(number=w341) -> (double precision float=w342:dbl)
            n259 = Subtract(x=w342, y=w336) -> (x-y=→"x-y 5":dbl)
            n260 = global read "Robot Global Data.vi" "Shooter Stable?"() -> (w329:bool)
            n261 = And(x=w329, y=w331) -> (x .and. y?=w327:bool)
            "count 2" <- w327
            n262 = feedback-in #16(w329) -> ()
            n263 = feedback #16(TRUE ("Shooter Stable?")) -> (w332:bool)
            n264 = Get Date/Time In Seconds() -> (seconds since 1Jan1904=w339:timestamp)
            n265 = Greater?(x=w329, y=w332) -> (0:w328:bool)
            "Edge 2" <- w328
            n266 = Add(x=w336, y=w335) -> (x+y=w338:dbl)
            n267 = To Double Precision Float(number=w339) -> (double precision float=w340:dbl)
            n268 = Or(x=w328, y=w327) -> (x .or. y?=w326:bool)
            n269 = Greater Or Equal?(x=w340, y=w338) -> ()  [unwired: 1 out]
            n270 = Or(x=FALSE, y=w326) -> (x .or. y?=w337:bool)
            "Shooter Stable" <- w330
          }
        }
        frame #7 {
          # "Ensure Fire 'Button' has gone\nFalse (Pulse Stretcher complete)\nbefore attempting to Fire again."
          n271 = while {
            i -> [w346]
            stop <- w347 continue-if-true
            n272 = global read "Robot Global Data.vi" "Report Fire"() -> (w347:bool)
            n273 = Wait (ms)(milliseconds to wait=u32 10) -> ()  [unwired: 1 out]
            "Report" <- w346
          }
        }
        frame #8 {
          # "Fire"
          # "Will PRIME turn off too early, \nbefore ball has left the Shooter?"
          # "Fire Ball 2"
          n274 = while {
            tunnel: w349 -> [w353]
            i -> [w350]
            stop <- w351 continue-if-true
            n275 = Get Date/Time In Seconds() -> (seconds since 1Jan1904=w355:timestamp)
            n276 = global read "Robot Global Data.vi" "PRIME"() -> (w351:bool)
            n277 = To Double Precision Float(number=w355) -> (double precision float=w354:dbl)
            n278 = Subtract(x=w354, y=w353) -> (x-y=→"x-y 6":dbl)
            n279 = Wait (ms)(milliseconds to wait=u32 10) -> ()  [unwired: 1 out]
            "Fire" <- w350
          }
          n280 = global write "Robot Global Data.vi" "Op Button 5"(TRUE ("Op Button 5")) -> ()
        }
        frame #9 {
          n281 = disable-structure shown="Disabled" {
            disable-tunnel: w359 -> [w363 _]
            disable-tunnel: w358 -> [w362 _]
            disable-tunnel: w357 -> [w361 _]
            frame Disabled {
              # "Push Bridge Down"
              n282 = while {
                tunnel: w363 -> [w369]
                tunnel: w362 -> [w374]
                tunnel: "Bridge Timeout (sec)" -> [w368]
                stop <- w365 stop-if-true
                # "Timeout"
                n283 = Get Date/Time In Seconds() -> (seconds since 1Jan1904=w375:timestamp)
                n284 = call <vilib>:"WPI_DigitalInputGetValue.vi"("DigitalInputDevRef"=w374) -> ("Value"=w373:bool)  [unwired: 8 in, 2 out]
                n285 = Get Date/Time In Seconds() -> (seconds since 1Jan1904=w371:timestamp)
                n286 = To Double Precision Float(number=w375) -> (double precision float=w376:dbl)
                n287 = Add(x=w369, y=w368) -> (x+y=w370:dbl)
                n288 = Not(x=w373) -> (.not. x?=w366:bool)
                n289 = To Double Precision Float(number=w371) -> (double precision float=w372:dbl)
                n290 = Subtract(x=w376, y=w369) -> (x-y=→"x-y 14":dbl)
                n291 = Greater Or Equal?(x=w372, y=w370) -> (x >= y?=w367:bool)
                n292 = Or(x=w366, y=w367) -> (x .or. y?=w365:bool)
                n293 = Wait (ms)(milliseconds to wait=u32 10) -> ()  [unwired: 1 out]
              }
              n294 = call <vilib>:"WPI_RelaySet.vi"("RelayValue"=WPI_RelayValue."Reverse", "RelayDevRef"=w361) -> ()  [unwired: 8 in, 2 out]
            }
            frame Enabled {
            }
          }
        }
        frame #10 {
          # "Fire Conv Off"
          n295 = global write "Robot Global Data.vi" "Op Button 5"(FALSE ("Op Button 5")) -> ()
          n296 = call <vilib>:"WPI_GyroReset.vi"("GyroDevRef"=w380) -> ()  [unwired: 9 in, 2 out]
        }
        frame #11 {
          # "Primitive Drive Straight Capability"
          # "Drive Straight to Coop Bridge"
          n297 = global write "Robot Global Data.vi" "Shooter RPM Control"(w383) -> ()
          n298 = while {
            tunnel: w385 -> [w386]
            tunnel: w384 -> [w405]
            tunnel: w382 -> [w396]
            tunnel: w381 -> [w387]
            stop <- w407 stop-if-true
            n299 = Get Date/Time In Seconds() -> (seconds since 1Jan1904=w390:timestamp)
            n300 = call <vilib>:"WPI_GyroGetAngle.vi"("GyroDevRef"=w396) -> ("Angle"=w393:dbl)  [unwired: 7 in, 3 out]
            n301 = Bundle("setpoint"=0.0, "Angle"=w393) -> (→"RPM Control Response":cluster{"setpoint":dbl, "Angle":dbl})  [unwired: 1 out]
            n302 = To Double Precision Float(number=w390) -> (double precision float=w389:dbl)
            n303 = Subtract(x=w389, y=w387) -> (x-y=→"x-y 7":dbl)
            n304 = Bundle("Prop"="Prop", "Int"="Int", "Deriv"="Deriv") -> (w397:cluster{"Prop":dbl, "Int":dbl, "Deriv":dbl})  [unwired: 1 out]
            n305 = global read "Robot Global Data.vi" "Avg Wheel Encoder"() -> (w406:dbl)
            n306 = Bundle("x"=0.7, -0.7) -> (w400:cluster{"x":dbl, dbl})  [unwired: 1 out]
            n307 = call-poly <vilib>:"PID.vi"("output range"=w400, "PID gains"=w397, "process variable"=w393, "setpoint"=0.0) -> ("output"=w391:dbl)  [unwired: 2 in, 5 out]
            "PID Output" <- w391
            n308 = Subtract(x=w386, y=w391) -> ()  [unwired: 1 out]
            n309 = Greater Or Equal?(x=w406, y=w405) -> (x >= y?=w407:bool)
            n310 = global write "Robot Global Data.vi" "X Axis Drive Cmd"(w386) -> ()
            n311 = global write "Robot Global Data.vi" "Y Axis Drive Cmd"(w386) -> ()
            n312 = Wait (ms)(milliseconds to wait=u32 10) -> ()  [unwired: 1 out]
          }
        }
        frame #12 {
          # "Turn on Auto-Target"
          # "Stop Drive, Brake,\nand Start up all Conveyors"
          # "Requires State Machine for more than one Ball"
          n313 = disable-structure shown="Disabled" {
            frame Disabled {
              # "Mid Conv Forward"
              # "Lo Conv Forward"
              # "Intake On"
              # "Fire Conv On"
              n314 = global write "Robot Global Data.vi" "Op Button 5"(TRUE ("Op Button 5")) -> ()
              n315 = global write "Robot Global Data.vi" "Op Button 8"(TRUE ("Op Button 5")) -> ()
              n316 = global write "Robot Global Data.vi" "Op Button 2"(TRUE ("Op Button 5")) -> ()
              n317 = global write "Robot Global Data.vi" "Op Button 1"(TRUE ("Op Button 5")) -> ()
            }
            frame Enabled {
            }
          }
          n318 = global write "Robot Global Data.vi" "Dr Button 2"(FALSE ("Dr Button 5")) -> ()
          n319 = global write "Robot Global Data.vi" "Dr Button 1"(FALSE ("Dr Button 5")) -> ()
          n320 = global write "Robot Global Data.vi" "Collector State Machine"(TRUE ("Collector State Machine")) -> ()
          n321 = global write "Robot Global Data.vi" "Op Button 7"(TRUE ("Dr Button 5")) -> ()
          n322 = global write "Robot Global Data.vi" "X Axis Drive Cmd"(w409) -> ()
          n323 = global write "Robot Global Data.vi" "Y Axis Drive Cmd"(w409) -> ()
        }
        frame #13 {
          # "Wait for Ball to reach Prime"
          # "Look for Target"
          n324 = Get Date/Time In Seconds() -> (seconds since 1Jan1904=w417:timestamp)
          n325 = To Double Precision Float(number=w417) -> (double precision float=w418:dbl)
          n326 = while {
            tunnel: w418 -> [w431]
            i -> [w430]
            stop <- w420 stop-if-true
            w425 = 1.0 ("upper limit")
            n327 = global read "Robot Global Data.vi" "Target Angle"() -> (w427:dbl)
            n328 = feedback #17(0) -> (w435:i32)
            "State 4" <- w435
            n329 = feedback #18() -> (w432:dbl)  [unwired: 1 in]
            n330 = case shown="0, Default" w435 {
              tunnel: [w448 w459 w466 w473] -> w428
              tunnel: [0.0 0.5 -0.5 0.5] -> w434
              tunnel: [w445 w461 0.0 ("Turret Yaw") 0.0 ("Turret Yaw")] -> w433
              tunnel: w432 -> [_ w461 _ _]
              tunnel: w431 -> [w440 _ _ _]
              frame 0, Default {
                # "Engage Auto-Target\n(take turret to last known target bearing)"
                n331 = Add(x=w440, y=1.0) -> (x+y=w437:dbl)
                n332 = global read "Robot Global Data.vi" "Turret Stable?"() -> (w443:bool)
                "Turret Stable? 4" <- w443
                n333 = Get Date/Time In Seconds() -> (seconds since 1Jan1904=w442:timestamp)
                n334 = global write "Robot Global Data.vi" "Op Button 7"(TRUE ("Op Button 7")) -> ()
                n335 = To Double Precision Float(number=w442) -> (double precision float=w438:dbl)
                n336 = Greater Or Equal?(x=w438, y=w437) -> (x >= y?=w441:bool)
                n337 = Or(x=w441, y=w443) -> (x .or. y?=w444:bool)
                n338 = global read "Robot Global Data.vi" "Turret Yaw"() -> (w445:dbl)
                n339 = Select(t=1, s=w444, f=0) -> (s? t:f=w448:i32)
              }
              frame 1 {
                # "Seek CCW a bit"
                n340 = global read "Robot Global Data.vi" "Left_Limit"() -> (w451:bool)
                n341 = Subtract(x=w461, y=15.0) -> (x-y=w455:dbl)
                n342 = global read "Robot Global Data.vi" "Turret Yaw"() -> (w456:dbl)
                n343 = Less Or Equal?(x=w456, y=w455) -> (x <= y?=w453:bool)
                n344 = Or(x=w453, y=w451) -> (x .or. y?=w452:bool)
                n345 = global write "Robot Global Data.vi" "Op Button 7"(FALSE ("Op Button 7")) -> ()
                n346 = Select(t=2, s=w452, f=1) -> (s? t:f=w459:i32)
              }
              frame 2 {
                # "Search CW"
                n347 = global read "Robot Global Data.vi" "Right_Limit"() -> (w463:bool)
                n348 = Select(t=3, s=w463, f=2) -> (s? t:f=w466:i32)
              }
              frame 3 {
                # "Search CCW"
                n349 = global read "Robot Global Data.vi" "Left_Limit"() -> (w469:bool)
                n350 = Select(t=2, s=w469, f=3) -> (s? t:f=w473:i32)
              }
            }
            n351 = global write "Robot Global Data.vi" "Turret Yaw Joystick Command"(w434) -> ()
            n352 = feedback-in #17(w428) -> ()
            n353 = feedback-in #18(w433) -> ()
            n354 = Negate(x=w425) -> (-x=w426:dbl)
            n355 = In Range and Coerce(upper limit=w425, x=w427, lower limit=w426) -> (In Range?=w424:bool)  [unwired: 1 out]
            "In Range? 4" <- w424
            n356 = global read "Robot Global Data.vi" "Valid Target ?"() -> (w419:bool)
            n357 = global read "Robot Global Data.vi" "PRIME"() -> (w421:bool)
            n358 = call "Stable.vi"("Pulse Width (sec)"="Pulse Width (sec) 4", "Signal Input"=w424) -> ("Stable"=w422:bool)  [unwired: 9 in]
            n359 = Compound Arithmetic op=AND(w422, w421, w419) -> (w420:bool)
            n360 = Wait (ms)(milliseconds to wait=u32 10) -> ()  [unwired: 1 out]
            "Numeric 4" <- w430
          }
        }
        frame #14 {
          # "Stabilize Distance Measurement"
          n361 = Get Date/Time In Seconds() -> (seconds since 1Jan1904=w476:timestamp)
          n362 = To Double Precision Float(number=w476) -> (double precision float=w475:dbl)
          n363 = while {
            tunnel: w475 -> [w483]
            stop <- w486 stop-if-true
            n364 = global read "Robot Global Data.vi" "Target Distance"() -> (w488:dbl)
            n365 = Get Date/Time In Seconds() -> (seconds since 1Jan1904=w485:timestamp)
            n366 = To Double Precision Float(number=w485) -> (double precision float=w482:dbl)
            n367 = Add(x=w483, y=4.0) -> (x+y=w481:dbl)
            n368 = Greater Or Equal?(x=w482, y=w481) -> (x >= y?=w479:bool)
            n369 = feedback #19() -> (w493:dbl)  [unwired: 1 in]
            n370 = feedback-in #19(w488) -> ()
            n371 = feedback #20() -> (w494:dbl)  [unwired: 1 in]
            n372 = feedback-in #20(w493) -> ()
            n373 = feedback #21() -> (w495:dbl)  [unwired: 1 in]
            n374 = feedback-in #21(w494) -> ()
            n375 = feedback #22() -> (w496:dbl)  [unwired: 1 in]
            n376 = feedback-in #22(w495) -> ()
            n377 = Bundle("Target Distance"=w496, "Target Distance"=w495, "Target Distance"=w494, "Target Distance"=w493, "Target Distance"=w488) -> (w492:T15)  [unwired: 1 in]
            n378 = Cluster To Array(cluster=w492) -> (array=w491:dbl[])
            n379 = call <vilib>:"Std Deviation and Variance.vi"("X"=w491) -> ("standard deviation"=w487:dbl)  [unwired: 1 in, 2 out]
            n380 = Less Or Equal?(x=w487, y=0.3) -> (x <= y?=w480:bool)
            n381 = Wait (ms)(milliseconds to wait=u32 5) -> ()  [unwired: 1 out]
            n382 = Or(x=w480, y=w479) -> (x .or. y?=w486:bool)
          }
          n383 = global write "Robot Global Data.vi" "Turret Yaw Joystick Command"(0.0 ("Turret Yaw Joystick Command")) -> ()
          n384 = global write "Robot Global Data.vi" "Auto Target"(FALSE ("Auto Target")) -> ()
        }
        frame #15 {
          # "Compute Shooter RPM and set Control value"
          n385 = global read "Robot Global Data.vi" "Target Distance"() -> (w498:dbl)
          "Target Distance 3" <- w498
          n386 = global read "Robot Global Data.vi" "Personality"() -> (w497:string)
          n387 = call "Distance to RPM_V1.vi"("Personality"=w497, "Target Distance"=w498) -> ("Shooter RPM Control"=w499:dbl)  [unwired: 3 in]
          "RPM Control 3" <- w499
          n388 = global write "Robot Global Data.vi" "Shooter RPM Control"(w499) -> ()
        }
        frame #16 {
          n389 = while {
            tunnel: w500 -> [w501]
            stop <- FALSE stop-if-true
            # "Fire"
            n390 = global read "Robot Global Data.vi" "Shooter Stable?"() -> (w504:bool)
            n391 = global read "Robot Global Data.vi" "PRIME"() -> (w505:bool)
            n392 = global read "Robot Global Data.vi" "Target Angle"() -> (w507:dbl)
            n393 = Absolute Value(x=w507) -> (abs(x)=w506:dbl)
            n394 = Less Or Equal?(x=w506, y=w501) -> (x <= y?=w503:bool)
            n395 = Compound Arithmetic op=AND(w505, w504, w503) -> (w502:bool)
            n396 = global write "Robot Global Data.vi" "Op Button 5"(w502) -> ()
            n397 = Wait (ms)(milliseconds to wait=u32 10) -> ()  [unwired: 1 out]
          }
        }
      }
    }
    frame 2 {
      n398 = flat-sequence {
        tunnel: w518 -> [w526]
        tunnel: w519 -> [w527]
        tunnel: w516 -> [w523]
        tunnel: w510 -> [w521]
        tunnel: w516 -> [w528]
        tunnel: w517 -> [w547]
        tunnel: w515 -> [w549]
        tunnel: w514 -> [w563]
        tunnel: w513 -> [w574]
        tunnel: w512 -> [w594]
        tunnel: w511 -> [w610]
        frame #0 {
          # "Requires Collector State Machine to be\nInert in Autonomous"
          # "Initialize, start Shooter,\nand Aim Turret at Target"
          n399 = call <vilib>:"WPI_EncoderReset.vi"("EncoderDevRef"=w527) -> ()  [unwired: 9 in, 2 out]
          n400 = call <vilib>:"WPI_EncoderReset.vi"("EncoderDevRef"=w526) -> ()  [unwired: 9 in, 2 out]
          n401 = Get Date/Time In Seconds() -> (seconds since 1Jan1904=w525:timestamp)
          n402 = global write "Robot Global Data.vi" "Shooter RPM Control"(w521) -> ()
          n403 = global write "Robot Global Data.vi" "Op Button 8"(TRUE) -> ()
          n404 = To Double Precision Float(number=w525) -> (double precision float=w524:dbl)
          n405 = Subtract(x=w524, y=w523) -> (x-y=→"x-y 15":dbl)
        }
        frame #1 {
          # "May need to test for Ready & Stable,\notherwise may fire on control overshoot"
          # "Wait for Shooter to reach RPM"
          n406 = while {
            tunnel: w528 -> [w538]
            i -> [w535]
            stop <- w543 stop-if-true
            # "Do Nothing 'til Shooter is at speed"
            n407 = global read "Robot Global Data.vi" "Shooter RPM Response"() -> (w545:dbl)
            n408 = global read "Robot Global Data.vi" "Shooter Stable?"() -> (w532:bool)
            n409 = Greater Or Equal?(x=w535, y=25) -> (x >= y?=w533:bool)
            n410 = Get Date/Time In Seconds() -> (seconds since 1Jan1904=w539:timestamp)
            n411 = And(x=w532, y=w533) -> (x .and. y?=w531:bool)
            n412 = To Double Precision Float(number=w539) -> (double precision float=w540:dbl)
            n413 = feedback-in #23(w532) -> ()
            n414 = feedback #23(TRUE ("Shooter Stable?")) -> (w537:bool)
            n415 = Subtract(x=w540, y=w538) -> (x-y=→"x-y 16":dbl)
            n416 = Greater?(x=w532, y=w537) -> (0:w530:bool)
            n417 = Greater Or Equal?(x=w545, y=1000.0) -> (x >= y?=w542:bool)
            n418 = Or(x=w530, y=w531) -> (x .or. y?=w529:bool)
            n419 = Wait (ms)(milliseconds to wait=u32 10) -> ()  [unwired: 1 out]
            n420 = And(x=w542, y=w529) -> (x .and. y?=w543:bool)
            "A2: S1" <- w535
          }
        }
        frame #2 {
          n421 = global write "Robot Global Data.vi" "X Axis Drive Cmd"(w547) -> ()
          n422 = global write "Robot Global Data.vi" "Y Axis Drive Cmd"(w547) -> ()
        }
        frame #3 {
          # "Fire"
          # "Will PRIME turn off too early, \nbefore ball has left the Shooter?"
          # "Fire Ball 1"
          n423 = while {
            tunnel: w549 -> [w554]
            tunnel: "Ball 1 Timeout (sec) 2" -> [w559]
            i -> [w551]
            stop <- w558 stop-if-true
            # "Timeout"
            # "Conv C Speed\nAlso known as Fire"
            n424 = global read "Robot Global Data.vi" "PRIME"() -> (w557:bool)
            n425 = Wait (ms)(milliseconds to wait=u32 10) -> ()  [unwired: 1 out]
            n426 = Get Date/Time In Seconds() -> (seconds since 1Jan1904=w560:timestamp)
            n427 = Not(x=w557) -> (.not. x?=w556:bool)
            n428 = Add(x=w554, y=w559) -> (x+y=w561:dbl)
            n429 = To Double Precision Float(number=w560) -> (double precision float=w555:dbl)
            n430 = Or(x=FALSE, y=w556) -> (x .or. y?=w558:bool)
            n431 = Greater Or Equal?(x=w555, y=w561) -> ()  [unwired: 1 out]
            n432 = Subtract(x=w555, y=w554) -> (x-y=→"x-y 17":dbl)
            "A2: F1" <- w551
          }
          n433 = global write "Robot Global Data.vi" "Op Button 5"(TRUE ("Op Button 5")) -> ()
        }
        frame #4 {
          # "Re prime for Ball 2"
          n434 = while {
            tunnel: w563 -> [w565]
            i -> [w564]
            stop <- w569 stop-if-true
            n435 = disable-structure shown="Disabled" {
              frame Disabled {
                # "Fire"
                n436 = global write "Robot Global Data.vi" "Op Button 1"(TRUE ("Op Button 5")) -> ()
                n437 = global write "Robot Global Data.vi" "Op Button 5"(TRUE ("Op Button 5")) -> ()
              }
              frame Enabled {
              }
            }
            n438 = Get Date/Time In Seconds() -> (seconds since 1Jan1904=w568:timestamp)
            n439 = global read "Robot Global Data.vi" "PRIME"() -> (w569:bool)
            n440 = To Double Precision Float(number=w568) -> (double precision float=w567:dbl)
            n441 = Subtract(x=w567, y=w565) -> (x-y=→"x-y 18":dbl)
            n442 = Wait (ms)(milliseconds to wait=u32 10) -> ()  [unwired: 1 out]
            "A2: P2" <- w564
          }
        }
        frame #5 {
          # "Un-Fire"
          n443 = global write "Robot Global Data.vi" "Op Button 5"(FALSE ("Op Button 5")) -> ()
        }
        frame #6 {
          # "May need to test for Ready & Stable,\notherwise may fire on control overshoot"
          # "Stop Conveyors and Spin Up Shooter"
          # "Spin Up"
          # "Stop"
          n444 = while {
            tunnel: w574 -> [w586]
            i -> [w583]
            stop <- w580 stop-if-true
            # "Do Nothing 'til Shooter is at speed"
            n445 = global read "Robot Global Data.vi" "Shooter Stable?"() -> (w578:bool)
            n446 = Greater Or Equal?(x=w583, y=25) -> (x >= y?=w579:bool)
            n447 = Get Date/Time In Seconds() -> (seconds since 1Jan1904=w587:timestamp)
            n448 = And(x=w578, y=w579) -> (x .and. y?=w577:bool)
            n449 = To Double Precision Float(number=w587) -> (double precision float=w588:dbl)
            n450 = feedback-in #24(w578) -> ()
            n451 = feedback #24(TRUE ("Shooter Stable?")) -> (w585:bool)
            n452 = Subtract(x=w588, y=w586) -> (x-y=→"x-y 19":dbl)
            n453 = Greater?(x=w578, y=w585) -> (0:w581:bool)
            n454 = Or(x=w581, y=w577) -> (x .or. y?=w580:bool)
            n455 = Wait (ms)(milliseconds to wait=u32 10) -> ()  [unwired: 1 out]
            "A2: S2" <- w583
          }
          n456 = disable-structure shown="Disabled" {
            frame Disabled {
              n457 = global write "Robot Global Data.vi" "Op Button 5"(FALSE ("Op Button 5")) -> ()
              n458 = global write "Robot Global Data.vi" "Op Button 1"(FALSE ("Op Button 5")) -> ()
            }
            frame Enabled {
            }
          }
        }
        frame #7 {
          # "Ensure Fire 'Button' has gone\nFalse (Pulse Stretcher complete)\nbefore attempting to Fire again."
          n459 = while {
            stop <- w592 continue-if-true
            n460 = global read "Robot Global Data.vi" "Report Fire"() -> (w592:bool)
            n461 = Wait (ms)(milliseconds to wait=u32 10) -> ()  [unwired: 1 out]
          }
        }
        frame #8 {
          # "Will PRIME turn off too early, \nbefore ball has left the Shooter?"
          # "Fire Ball 2"
          n462 = while {
            tunnel: w594 -> [w599]
            tunnel: "Ball 2 Timeout (sec) 2" -> [w601]
            i -> [w596]
            stop <- w603 stop-if-true
            n463 = Wait (ms)(milliseconds to wait=u32 10) -> ()  [unwired: 1 out]
            n464 = global read "Robot Global Data.vi" "PRIME"() -> (w604:bool)
            n465 = Get Date/Time In Seconds() -> (seconds since 1Jan1904=w605:timestamp)
            n466 = Add(x=w599, y=w601) -> (x+y=w606:dbl)
            n467 = To Double Precision Float(number=w605) -> (double precision float=w600:dbl)
            n468 = Not(x=w604) -> (.not. x?=w602:bool)
            n469 = Or(x=FALSE, y=w602) -> (x .or. y?=w603:bool)
            n470 = Greater Or Equal?(x=w600, y=w606) -> ()  [unwired: 1 out]
            n471 = Subtract(x=w600, y=w599) -> (x-y=→"x-y 20":dbl)
            "A2: F2" <- w596
          }
          n472 = global write "Robot Global Data.vi" "Op Button 5"(TRUE ("Op Button 5")) -> ()
        }
        frame #9 {
          # "Don't Turn on Auto-Target"
          n473 = global write "Robot Global Data.vi" "Collector State Machine"(TRUE ("Collector State Machine")) -> ()
          n474 = global write "Robot Global Data.vi" "Op Button 5"(FALSE ("Op Button 5")) -> ()
          n475 = global write "Robot Global Data.vi" "Op Button 7"(FALSE ("Dr Button 5")) -> ()
          n476 = call <vilib>:"WPI_RelaySet.vi"("RelayValue"=WPI_RelayValue."Off", "RelayDevRef"=w610) -> ()  [unwired: 8 in, 2 out]
        }
        frame #10 {
          # "Ensure Fire 'Button' has gone\nFalse (Pulse Stretcher complete)\nbefore attempting to Fire again."
          n477 = while {
            stop <- w614 continue-if-true
            n478 = global read "Robot Global Data.vi" "Report Fire"() -> (w614:bool)
            n479 = Wait (ms)(milliseconds to wait=u32 10) -> ()  [unwired: 1 out]
          }
        }
        frame #11 {
          n480 = while {
            i -> [w623]
            stop <- FALSE stop-if-true
            n481 = global read "Robot Global Data.vi" "Shooter Stable?"() -> (w618:bool)
            n482 = global read "Robot Global Data.vi" "PRIME"() -> (w625:bool)
            n483 = Greater Or Equal?(x=w623, y=25) -> (x >= y?=w621:bool)
            n484 = And(x=w618, y=w621) -> (x .and. y?=w616:bool)
            n485 = feedback-in #25(w618) -> ()
            n486 = feedback #25(TRUE ("Shooter Stable?")) -> (w619:bool)
            n487 = Greater?(x=w618, y=w619) -> (0:w617:bool)
            n488 = Or(x=w617, y=w616) -> (x .or. y?=w615:bool)
            n489 = And(x=w625, y=w615) -> (x .and. y?=w624:bool)
            n490 = global write "Robot Global Data.vi" "Op Button 5"(w624) -> ()
            n491 = Wait (ms)(milliseconds to wait=u32 10) -> ()  [unwired: 1 out]
          }
        }
      }
    }
    frame 3 {
      n492 = global write "Robot Global Data.vi" "Collector State Machine"(FALSE ("Shooter Ready?")) -> ()
      n493 = flat-sequence {
        tunnel: w637 -> [w644]
        tunnel: w638 -> [w645]
        tunnel: w636 -> [w646]
        tunnel: w630 -> [w640]
        tunnel: w630 -> [w647]
        tunnel: w635 -> [w666]
        tunnel: w634 -> [w670]
        tunnel: w630 -> [w672]
        tunnel: w633 -> [w686]
        tunnel: w632 -> [w694]
        tunnel: w629 -> [w714]
        tunnel: w631 -> [w729]
        frame #0 {
          # "Requires Collector State Machine to be\nInert in Autonomous"
          # "Initialize, start Shooter,\nand Aim Turret at Target"
          n494 = call <vilib>:"WPI_EncoderReset.vi"("EncoderDevRef"=w645) -> ()  [unwired: 9 in, 2 out]
          n495 = call <vilib>:"WPI_EncoderReset.vi"("EncoderDevRef"=w644) -> ()  [unwired: 9 in, 2 out]
          n496 = Get Date/Time In Seconds() -> (seconds since 1Jan1904=w643:timestamp)
          n497 = global write "Robot Global Data.vi" "Shooter RPM Control"(w646) -> ()
          n498 = global write "Robot Global Data.vi" "Op Button 1"(FALSE ("Op Button 5")) -> ()
          n499 = To Double Precision Float(number=w643) -> (double precision float=w642:dbl)
          n500 = Subtract(x=w642, y=w640) -> (x-y=→"x-y 21":dbl)
        }
        frame #1 {
          # "May need to test for Ready & Stable,\notherwise may fire on control overshoot"
          # "Wait for Shooter to reach RPM"
          n501 = while {
            tunnel: w647 -> [w657]
            i -> [w656]
            stop <- w662 stop-if-true
            # "Do Nothing 'til Shooter is at speed"
            n502 = global read "Robot Global Data.vi" "Shooter RPM Response"() -> (w664:dbl)
            n503 = global read "Robot Global Data.vi" "Shooter Stable?"() -> (w649:bool)
            n504 = Greater Or Equal?(x=w656, y=25) -> (x >= y?=w650:bool)
            n505 = And(x=w649, y=w650) -> (x .and. y?=w648:bool)
            n506 = feedback-in #26(w649) -> ()
            n507 = feedback #26(TRUE ("Shooter Stable?")) -> (w654:bool)
            n508 = Get Date/Time In Seconds() -> (seconds since 1Jan1904=w658:timestamp)
            n509 = Greater Or Equal?(x=w664, y=1000.0) -> (x >= y?=w661:bool)
            n510 = Greater?(x=w649, y=w654) -> (0:w652:bool)
            n511 = Wait (ms)(milliseconds to wait=u32 10) -> ()  [unwired: 1 out]
            n512 = To Double Precision Float(number=w658) -> (double precision float=w659:dbl)
            n513 = Or(x=w652, y=w648) -> (x .or. y?=w651:bool)
            n514 = Subtract(x=w659, y=w657) -> (x-y=→"x-y 22":dbl)
            n515 = And(x=w661, y=w651) -> (x .and. y?=w662:bool)
          }
        }
        frame #2 {
          n516 = global write "Robot Global Data.vi" "X Axis Drive Cmd"(w666) -> ()
          n517 = global write "Robot Global Data.vi" "Y Axis Drive Cmd"(w666) -> ()
        }
        frame #3 {
          n518 = To Long Integer(number=w670) -> (32bit integer=w669:i32)
          n519 = Multiply(x=w669, y=1000) -> (x*y=w667:i32)
          n520 = Wait (ms)(milliseconds to wait=w667) -> ()  [unwired: 1 out]
        }
        frame #4 {
          # "Fire"
          # "Will PRIME turn off too early, \nbefore ball has left the Shooter?"
          # "Fire Ball 1"
          n521 = while {
            tunnel: "Ball 1 Timeout (sec) 3" -> [w681]
            tunnel: w672 -> [w674]
            stop <- w680 stop-if-true
            # "Timeout"
            n522 = global read "Robot Global Data.vi" "PRIME"() -> (w679:bool)
            n523 = Wait (ms)(milliseconds to wait=u32 10) -> ()  [unwired: 1 out]
            n524 = Get Date/Time In Seconds() -> (seconds since 1Jan1904=w682:timestamp)
            n525 = Not(x=w679) -> (.not. x?=w677:bool)
            n526 = Add(x=w674, y=w681) -> (x+y=w683:dbl)
            n527 = To Double Precision Float(number=w682) -> (double precision float=w676:dbl)
            n528 = Greater Or Equal?(x=w676, y=w683) -> (x >= y?=w678:bool)
            n529 = Or(x=w678, y=w677) -> (x .or. y?=w680:bool)
            n530 = Subtract(x=w676, y=w674) -> (x-y=→"x-y 23":dbl)
          }
          n531 = global write "Robot Global Data.vi" "Op Button 5"(TRUE ("Op Button 5")) -> ()
        }
        frame #5 {
          # "Fire"
          # "Re prime for Ball 2"
          n532 = while {
            tunnel: w686 -> [w689]
            stop <- w688 stop-if-true
            n533 = Get Date/Time In Seconds() -> (seconds since 1Jan1904=w692:timestamp)
            n534 = global read "Robot Global Data.vi" "PRIME"() -> (w688:bool)
            n535 = To Double Precision Float(number=w692) -> (double precision float=w691:dbl)
            n536 = Subtract(x=w691, y=w689) -> (x-y=→"x-y 24":dbl)
            n537 = Wait (ms)(milliseconds to wait=u32 10) -> ()  [unwired: 1 out]
          }
          n538 = disable-structure shown="Disabled" {
            frame Disabled {
              n539 = global write "Robot Global Data.vi" "Op Button 1"(TRUE ("Op Button 5")) -> ()
            }
            frame Enabled {
            }
          }
          n540 = global write "Robot Global Data.vi" "Op Button 5"(FALSE ("Op Button 5")) -> ()
        }
        frame #6 {
          # "May need to test for Ready & Stable,\notherwise may fire on control overshoot"
          # "Stop Conveyors and Spin Up Shooter"
          # "Spin Up"
          # "Stop"
          n541 = while {
            tunnel: w694 -> [w706]
            i -> [w703]
            stop <- w697 stop-if-true
            # "Do Nothing 'til Shooter is at speed"
            n542 = global read "Robot Global Data.vi" "Shooter Stable?"() -> (w700:bool)
            "Shooter Ready? 4" <- w700
            n543 = Greater Or Equal?(x=w703, y=25) -> (x >= y?=w705:bool)
            n544 = Get Date/Time In Seconds() -> (seconds since 1Jan1904=w707:timestamp)
            n545 = And(x=w700, y=w705) -> (x .and. y?=w698:bool)
            n546 = To Double Precision Float(number=w707) -> (double precision float=w708:dbl)
            n547 = feedback #27(TRUE ("PRIME")) -> (w701:bool)
            n548 = feedback-in #27(w700) -> ()
            n549 = Subtract(x=w708, y=w706) -> (x-y=→"x-y 25":dbl)
            n550 = Greater?(x=w700, y=w701) -> (0:w699:bool)
            n551 = Or(x=w699, y=w698) -> (x .or. y?=w697:bool)
            n552 = Wait (ms)(milliseconds to wait=u32 10) -> ()  [unwired: 1 out]
          }
          n553 = disable-structure shown="Disabled" {
            frame Disabled {
              n554 = global write "Robot Global Data.vi" "Op Button 5"(FALSE ("Op Button 5")) -> ()
              n555 = global write "Robot Global Data.vi" "Op Button 1"(FALSE ("Op Button 5")) -> ()
            }
            frame Enabled {
            }
          }
        }
        frame #7 {
          # "Ensure Fire 'Button' has gone\nFalse (Pulse Stretcher complete)\nbefore attempting to Fire again."
          n556 = while {
            stop <- w712 continue-if-true
            n557 = global read "Robot Global Data.vi" "Report Fire"() -> (w712:bool)
            n558 = Wait (ms)(milliseconds to wait=u32 10) -> ()  [unwired: 1 out]
          }
        }
        frame #8 {
          # "Will PRIME turn off too early, \nbefore ball has left the Shooter?"
          # "Fire Ball 2"
          n559 = while {
            tunnel: "Ball 2 Timeout (sec) 3" -> [w719]
            tunnel: w714 -> [w716]
            stop <- w722 stop-if-true
            n560 = Wait (ms)(milliseconds to wait=u32 10) -> ()  [unwired: 1 out]
            n561 = global read "Robot Global Data.vi" "PRIME"() -> (w723:bool)
            n562 = Get Date/Time In Seconds() -> (seconds since 1Jan1904=w724:timestamp)
            n563 = Add(x=w716, y=w719) -> (x+y=w725:dbl)
            n564 = To Double Precision Float(number=w724) -> (double precision float=w718:dbl)
            n565 = Not(x=w723) -> (.not. x?=w721:bool)
            n566 = Greater Or Equal?(x=w718, y=w725) -> (x >= y?=w720:bool)
            n567 = Or(x=w720, y=w721) -> (x .or. y?=w722:bool)
            n568 = Subtract(x=w718, y=w716) -> (x-y=→"x-y 26":dbl)
          }
          n569 = global write "Robot Global Data.vi" "Op Button 5"(TRUE ("Op Button 5")) -> ()
        }
        frame #9 {
          # "Turn on Auto-Target"
          n570 = disable-structure shown="Disabled" {
            frame Disabled {
              n571 = global write "Robot Global Data.vi" "Collector State Machine"(TRUE ("Collector State Machine")) -> ()
            }
            frame Enabled {
            }
          }
          n572 = global write "Robot Global Data.vi" "Op Button 7"(TRUE ("Dr Button 5")) -> ()
          n573 = disable-structure shown="Disabled" {
            frame Disabled {
              n574 = Wait (ms)(milliseconds to wait=u32 5000) -> ()  [unwired: 1 out]
            }
            frame Enabled {
            }
          }
          n575 = global write "Robot Global Data.vi" "Op Button 5"(FALSE ("Op Button 5")) -> ()
          n576 = call <vilib>:"WPI_RelaySet.vi"("RelayValue"=WPI_RelayValue."Off", "RelayDevRef"=w729) -> ()  [unwired: 8 in, 2 out]
        }
        frame #10 {
          # "Ensure Fire 'Button' has gone\nFalse (Pulse Stretcher complete)\nbefore attempting to Fire again."
          n577 = while {
            stop <- w734 continue-if-true
            n578 = global read "Robot Global Data.vi" "Report Fire"() -> (w734:bool)
            n579 = Wait (ms)(milliseconds to wait=u32 10) -> ()  [unwired: 1 out]
          }
        }
        frame #11 {
          n580 = while {
            i -> [w743]
            stop <- FALSE stop-if-true
            n581 = global read "Robot Global Data.vi" "Shooter Stable?"() -> (w737:bool)
            n582 = global read "Robot Global Data.vi" "PRIME"() -> (w745:bool)
            n583 = Greater Or Equal?(x=w743, y=25) -> (x >= y?=w741:bool)
            n584 = feedback-in #28(w737) -> ()
            n585 = feedback #28(TRUE ("Shooter Stable?")) -> (w738:bool)
            n586 = And(x=w737, y=w741) -> (x .and. y?=w740:bool)
            n587 = Greater?(x=w737, y=w738) -> (0:w736:bool)
            n588 = Or(x=w736, y=w740) -> (x .or. y?=w735:bool)
            n589 = And(x=w745, y=w735) -> (x .and. y?=w744:bool)
            n590 = global write "Robot Global Data.vi" "Op Button 5"(w744) -> ()
            n591 = Wait (ms)(milliseconds to wait=u32 10) -> ()  [unwired: 1 out]
          }
        }
      }
    }
    frame 4 {
      n592 = flat-sequence {
        tunnel: w756 -> [w769]
        tunnel: w757 -> [w770]
        tunnel: w758 -> [w771]
        tunnel: w754 -> [w766]
        tunnel: w754 -> [w774]
        tunnel: w755 -> [w799]
        tunnel: w749 -> [w800]
        tunnel: w753 -> [w805]
        tunnel: w752 -> [w813]
        tunnel: w750 -> [w823]
        tunnel: w750 -> [w849]
        tunnel: w759 -> [w856]
        tunnel: w750 -> [w858]
        tunnel: w762 -> [w859]
        tunnel: w763 -> [w860]
        tunnel: w760 -> [w861]
        tunnel: w761 -> [w862]
        tunnel: w751 -> [w886]
        tunnel: w750 -> [_]
        tunnel: w748 -> [w899]
        frame #0 {
          # "Requires Collector State Machine to be\nInert in Autonomous"
          # "Initialize, start Shooter,\nand Aim Turret at Target"
          n593 = call <vilib>:"WPI_EncoderReset.vi"("EncoderDevRef"=w770) -> ()  [unwired: 9 in, 2 out]
          n594 = call <vilib>:"WPI_EncoderReset.vi"("EncoderDevRef"=w769) -> ()  [unwired: 9 in, 2 out]
          n595 = Get Date/Time In Seconds() -> (seconds since 1Jan1904=w768:timestamp)
          n596 = To Double Precision Float(number=w768) -> (double precision float=w767:dbl)
          n597 = disable-structure shown="Disabled" {
            frame Disabled {
              n598 = global write "Robot Global Data.vi" "Op Button 1"(FALSE ("Op Button 5")) -> ()
            }
            frame Enabled {
            }
          }
          n599 = Subtract(x=w767, y=w766) -> (x-y=→"x-y 27":dbl)
          n600 = global write "Robot Global Data.vi" "Shooter RPM Control"(w771) -> ()
          n601 = global write "Robot Global Data.vi" "Dr Button 2"(TRUE ("Dr Button 5")) -> ()
        }
        frame #1 {
          # "May need to test for Ready & Stable,\notherwise may fire on control overshoot"
          # "Wait for Shooter to reach RPM"
          n602 = while {
            tunnel: w774 -> [w785]
            tunnel: "Ball 1 Timeout (sec) 4" -> [w786]
            i -> [w782]
            stop <- w791 stop-if-true
            # "Timeout"
            # "Do Nothing 'til Shooter is at speed"
            n603 = global read "Robot Global Data.vi" "Shooter RPM Response"() -> (w797:dbl)
            n604 = global read "Robot Global Data.vi" "Shooter Stable?"() -> (w776:bool)
            n605 = Greater Or Equal?(x=w782, y=25) -> (x >= y?=w777:bool)
            n606 = And(x=w776, y=w777) -> (x .and. y?=w775:bool)
            n607 = feedback-in #29(w776) -> ()
            n608 = feedback #29(TRUE ("Shooter Stable?")) -> (w783:bool)
            n609 = Get Date/Time In Seconds() -> (seconds since 1Jan1904=w792:timestamp)
            n610 = Greater Or Equal?(x=w797, y=1000.0) -> (x >= y?=w795:bool)
            n611 = Greater?(x=w776, y=w783) -> (0:w780:bool)
            n612 = To Double Precision Float(number=w792) -> (double precision float=w793:dbl)
            n613 = Or(x=w780, y=w775) -> (x .or. y?=w778:bool)
            n614 = Wait (ms)(milliseconds to wait=u32 10) -> ()  [unwired: 1 out]
            n615 = And(x=w795, y=w778) -> (x .and. y?=w787:bool)
            n616 = Subtract(x=w793, y=w785) -> (x-y=→"x-y 28":dbl)
            n617 = Or(x=FALSE, y=w787) -> (x .or. y?=w791:bool)
            n618 = Get Date/Time In Seconds() -> (seconds since 1Jan1904=w789:timestamp)
            n619 = Add(x=w785, y=w786) -> (x+y=w788:dbl)
            n620 = To Double Precision Float(number=w789) -> (double precision float=w790:dbl)
            n621 = Greater Or Equal?(x=w790, y=w788) -> ()  [unwired: 1 out]
          }
        }
        frame #2 {
          n622 = global write "Robot Global Data.vi" "X Axis Drive Cmd"(w799) -> ()
          n623 = global write "Robot Global Data.vi" "Y Axis Drive Cmd"(w799) -> ()
        }
        frame #3 {
          n624 = To Long Integer(number=w800) -> (32bit integer=w803:i32)
          n625 = Multiply(x=w803, y=1000) -> (x*y=w801:i32)
          n626 = Wait (ms)(milliseconds to wait=w801) -> ()  [unwired: 1 out]
        }
        frame #4 {
          # "Fire"
          # "Will PRIME turn off too early, \nbefore ball has left the Shooter?"
          # "Fire Ball 1"
          n627 = while {
            tunnel: w805 -> [w808]
            stop <- w806 continue-if-true
            n628 = global read "Robot Global Data.vi" "PRIME"() -> (w806:bool)
            n629 = Get Date/Time In Seconds() -> (seconds since 1Jan1904=w810:timestamp)
            n630 = To Double Precision Float(number=w810) -> (double precision float=w809:dbl)
            n631 = Subtract(x=w809, y=w808) -> (x-y=→"x-y 29":dbl)
            n632 = Wait (ms)(milliseconds to wait=u32 10) -> ()  [unwired: 1 out]
          }
          n633 = global write "Robot Global Data.vi" "Op Button 5"(TRUE ("Op Button 5")) -> ()
        }
        frame #5 {
          # "Re prime for Ball 2"
          n634 = while {
            tunnel: w813 -> [w816]
            stop <- w820 stop-if-true
            n635 = Get Date/Time In Seconds() -> (seconds since 1Jan1904=w819:timestamp)
            n636 = To Double Precision Float(number=w819) -> (double precision float=w818:dbl)
            n637 = global read "Robot Global Data.vi" "PRIME"() -> (w820:bool)
            n638 = Subtract(x=w818, y=w816) -> (x-y=→"x-y 30":dbl)
            n639 = Wait (ms)(milliseconds to wait=u32 10) -> ()  [unwired: 1 out]
          }
          n640 = disable-structure shown="Disabled" {
            frame Disabled {
              # "Mid Conv Forward"
              # "Fire Conv On"
              n641 = global write "Robot Global Data.vi" "Op Button 1"(TRUE ("Op Button 5")) -> ()
              n642 = global write "Robot Global Data.vi" "Op Button 5"(TRUE ("Op Button 5")) -> ()
            }
            frame Enabled {
            }
          }
          n643 = global write "Robot Global Data.vi" "Op Button 5"(FALSE ("Op Button 5")) -> ()
        }
        frame #6 {
          # "May need to test for Ready & Stable,\notherwise may fire on control overshoot"
          # "Stop Conveyors and Spin Up Shooter"
          # "Spin Up"
          # "Stop"
          n644 = disable-structure shown="Disabled" {
            frame Disabled {
              # "Mid Conv Off"
              # "Fire Conv Off"
              n645 = global write "Robot Global Data.vi" "Op Button 5"(FALSE ("Op Button 5")) -> ()
              n646 = global write "Robot Global Data.vi" "Op Button 1"(FALSE ("Op Button 5")) -> ()
            }
            frame Enabled {
            }
          }
          n647 = while {
            tunnel: w823 -> [w836]
            tunnel: "Ball 2 Timeout (sec) 4" -> [w835]
            i -> [w834]
            stop <- w837 stop-if-true
            # "Timeout"
            # "Do Nothing 'til Shooter is at speed"
            n648 = global read "Robot Global Data.vi" "Shooter Stable?"() -> (w829:bool)
            n649 = Greater Or Equal?(x=w834, y=25) -> (x >= y?=w832:bool)
            n650 = Wait (ms)(milliseconds to wait=u32 10) -> ()  [unwired: 1 out]
            n651 = And(x=w829, y=w832) -> (x .and. y?=w827:bool)
            n652 = feedback-in #30(w829) -> ()
            n653 = feedback #30(TRUE ("Shooter Stable?")) -> (w830:bool)
            n654 = Greater?(x=w829, y=w830) -> (0:w828:bool)
            n655 = Get Date/Time In Seconds() -> (seconds since 1Jan1904=w842:timestamp)
            n656 = To Double Precision Float(number=w842) -> (double precision float=w843:dbl)
            n657 = Or(x=w828, y=w827) -> (x .or. y?=w826:bool)
            n658 = Subtract(x=w843, y=w836) -> (x-y=→"x-y 31":dbl)
            n659 = Get Date/Time In Seconds() -> (seconds since 1Jan1904=w840:timestamp)
            n660 = Add(x=w836, y=w835) -> (x+y=w839:dbl)
            n661 = To Double Precision Float(number=w840) -> (double precision float=w841:dbl)
            n662 = Greater Or Equal?(x=w841, y=w839) -> (x >= y?=w838:bool)
            n663 = Or(x=w838, y=w826) -> (x .or. y?=w837:bool)
          }
        }
        frame #7 {
          # "Ensure Fire 'Button' has gone\nFalse (Pulse Stretcher complete)\nbefore attempting to Fire again."
          n664 = while {
            stop <- w847 continue-if-true
            n665 = global read "Robot Global Data.vi" "Report Fire"() -> (w847:bool)
            n666 = Wait (ms)(milliseconds to wait=u32 10) -> ()  [unwired: 1 out]
          }
        }
        frame #8 {
          # "Fire"
          # "Will PRIME turn off too early, \nbefore ball has left the Shooter?"
          # "Fire Ball 2"
          n667 = while {
            tunnel: w849 -> [w852]
            stop <- w850 continue-if-true
            n668 = Get Date/Time In Seconds() -> (seconds since 1Jan1904=w854:timestamp)
            n669 = global read "Robot Global Data.vi" "PRIME"() -> (w850:bool)
            n670 = To Double Precision Float(number=w854) -> (double precision float=w853:dbl)
            n671 = Subtract(x=w853, y=w852) -> (x-y=→"x-y 32":dbl)
            n672 = Wait (ms)(milliseconds to wait=u32 10) -> ()  [unwired: 1 out]
          }
          n673 = global write "Robot Global Data.vi" "Op Button 5"(TRUE ("Op Button 5")) -> ()
        }
        frame #9 {
          # "Fire Conv Off"
          n674 = global write "Robot Global Data.vi" "Op Button 5"(FALSE ("Op Button 5")) -> ()
          n675 = call <vilib>:"WPI_GyroReset.vi"("GyroDevRef"=w856) -> ()  [unwired: 9 in, 2 out]
        }
        frame #10 {
          # "Primitive Drive Straight Capability"
          # "Drive Straight to Coop Bridge"
          n676 = global write "Robot Global Data.vi" "Shooter RPM Control"(w860) -> ()
          n677 = while {
            tunnel: w862 -> [w863]
            tunnel: w861 -> [w882]
            tunnel: w859 -> [w873]
            tunnel: w858 -> [w864]
            stop <- w884 stop-if-true
            n678 = call <vilib>:"WPI_GyroGetAngle.vi"("GyroDevRef"=w873) -> ("Angle"=w870:dbl)  [unwired: 7 in, 3 out]
            n679 = Bundle("setpoint"=0.0, "Angle"=w870) -> (→"RPM Control Response 2":cluster{"setpoint":dbl, "Angle":dbl})  [unwired: 1 out]
            n680 = Get Date/Time In Seconds() -> (seconds since 1Jan1904=w867:timestamp)
            n681 = To Double Precision Float(number=w867) -> (double precision float=w866:dbl)
            n682 = Subtract(x=w866, y=w864) -> (x-y=→"x-y 34":dbl)
            n683 = Bundle("Prop 2"="Prop 2", "Int 2"="Int 2", "Deriv 2"="Deriv 2") -> (w874:T16)  [unwired: 1 out]
            n684 = global read "Robot Global Data.vi" "Avg Wheel Encoder"() -> (w883:dbl)
            n685 = Bundle("x"=0.7, -0.7) -> (w877:cluster{"x":dbl, dbl})  [unwired: 1 out]
            n686 = call-poly <vilib>:"PID.vi"("output range"=w877, "PID gains"=w874, "process variable"=w870, "setpoint"=0.0) -> ("output"=w868:dbl)  [unwired: 2 in, 5 out]
            "PID Output 2" <- w868
            n687 = Subtract(x=w863, y=w868) -> ()  [unwired: 1 out]
            n688 = Greater Or Equal?(x=w883, y=w882) -> (x >= y?=w884:bool)
            n689 = global write "Robot Global Data.vi" "X Axis Drive Cmd"(w863) -> ()
            n690 = global write "Robot Global Data.vi" "Y Axis Drive Cmd"(w863) -> ()
            n691 = Wait (ms)(milliseconds to wait=u32 10) -> ()  [unwired: 1 out]
          }
        }
        frame #11 {
          # "Turn on Auto-Target"
          # "Stop Drive, Brake,\nand Start up all Conveyors"
          # "Requires State Machine for more than one Ball"
          n692 = disable-structure shown="Disabled" {
            frame Disabled {
              # "Mid Conv Forward"
              # "Lo Conv Forward"
              # "Intake On"
              # "Fire Conv On"
              n693 = global write "Robot Global Data.vi" "Op Button 5"(TRUE ("Op Button 5")) -> ()
              n694 = global write "Robot Global Data.vi" "Op Button 8"(TRUE ("Op Button 5")) -> ()
              n695 = global write "Robot Global Data.vi" "Op Button 2"(TRUE ("Op Button 5")) -> ()
              n696 = global write "Robot Global Data.vi" "Op Button 1"(TRUE ("Op Button 5")) -> ()
            }
            frame Enabled {
            }
          }
          n697 = global write "Robot Global Data.vi" "Dr Button 1"(FALSE ("Dr Button 5")) -> ()
          n698 = global write "Robot Global Data.vi" "Dr Button 2"(FALSE ("Dr Button 5")) -> ()
          n699 = global write "Robot Global Data.vi" "Collector State Machine"(TRUE ("Collector State Machine")) -> ()
          n700 = global write "Robot Global Data.vi" "Op Button 7"(TRUE ("Dr Button 5")) -> ()
          n701 = global write "Robot Global Data.vi" "X Axis Drive Cmd"(w886) -> ()
          n702 = global write "Robot Global Data.vi" "Y Axis Drive Cmd"(w886) -> ()
        }
        frame #12 {
          # "Ensure Fire 'Button' has gone\nFalse (Pulse Stretcher complete)\nbefore attempting to Fire again."
          n703 = while {
            stop <- w895 continue-if-true
            n704 = global read "Robot Global Data.vi" "Report Fire"() -> (w895:bool)
            n705 = Wait (ms)(milliseconds to wait=u32 10) -> ()  [unwired: 1 out]
          }
        }
        frame #13 {
          n706 = while {
            stop <- FALSE stop-if-true
            # "Fire"
            n707 = global read "Robot Global Data.vi" "PRIME"() -> (w896:bool)
            n708 = global write "Robot Global Data.vi" "Op Button 5"(w896) -> ()
            n709 = Wait (ms)(milliseconds to wait=u32 10) -> ()  [unwired: 1 out]
          }
        }
        frame #14 {
          n710 = while {
            tunnel: w899 -> [w900]
            stop <- FALSE stop-if-true
            # "Fire"
            n711 = global read "Robot Global Data.vi" "Shooter Stable?"() -> (w903:bool)
            n712 = global read "Robot Global Data.vi" "PRIME"() -> (w904:bool)
            n713 = global read "Robot Global Data.vi" "Target Angle"() -> (w906:dbl)
            n714 = Absolute Value(x=w906) -> (abs(x)=w905:dbl)
            n715 = Less Or Equal?(x=w905, y=w900) -> (x <= y?=w902:bool)
            n716 = Compound Arithmetic op=AND(w904, w903, w902) -> (w901:bool)
            n717 = global write "Robot Global Data.vi" "Op Button 5"(w901) -> ()
            n718 = Wait (ms)(milliseconds to wait=u32 10) -> ()  [unwired: 1 out]
          }
        }
      }
    }
    frame 5 {
      n719 = flat-sequence {
        tunnel: w924 -> [w929]
        tunnel: w925 -> [w930]
        tunnel: [w930] -> w912
        tunnel: [w929] -> w911
        tunnel: w922 -> [_]
        tunnel: w921 -> [_]
        tunnel: w917 -> [_]
        tunnel: w914 -> [w927]
        tunnel: w912 -> [w932]
        tunnel: w911 -> [w931]
        tunnel: w920 -> [w934]
        tunnel: w920 -> [w939]
        tunnel: w919 -> [w938]
        tunnel: w918 -> [w937]
        tunnel: w917 -> [w936]
        tunnel: w913 -> [w962]
        tunnel: w916 -> [w1051]
        tunnel: w909 -> [w1050]
        tunnel: w916 -> [w1073]
        tunnel: w915 -> [w1093]
        tunnel: w909 -> [w1091]
        tunnel: w923 -> [w1120]
        tunnel: w915 -> [w1124]
        tunnel: w910 -> [w1135]
        frame #0 {
          # "Intake Off"
          # "Bridge Down"
          n720 = global write "Robot Global Data.vi" "Dr Button 2"(TRUE ("Dr Button 5")) -> ()
          n721 = global write "Robot Global Data.vi" "Op Button 8"(TRUE ("Dr Button 5")) -> ()
          n722 = global write "Robot Global Data.vi" "Shooter RPM Control"(w927) -> ()
        }
        frame #1 {
          n723 = call <vilib>:"WPI_EncoderReset.vi"("EncoderDevRef"=w931) -> ()  [unwired: 9 in, 2 out]
          n724 = call <vilib>:"WPI_EncoderReset.vi"("EncoderDevRef"=w932) -> ()  [unwired: 9 in, 2 out]
        }
        frame #2 {
          # "Turn on Auto-Target"
          # "Fire Conv Off"
          n725 = global write "Robot Global Data.vi" "Op Button 5"(FALSE ("Op Button 5")) -> ()
          n726 = global write "Robot Global Data.vi" "Op Button 7"(TRUE ("Dr Button 5")) -> ()
          n727 = call <vilib>:"WPI_GyroReset.vi"("GyroDevRef"=w934) -> ()  [unwired: 9 in, 2 out]
        }
        frame #3 {
          # "Primitive Drive Straight Capability"
          # "Drive Straight to Coop Bridge"
          n728 = while {
            tunnel: w938 -> [w940]
            tunnel: w937 -> [w959]
            tunnel: w939 -> [w950]
            tunnel: w936 -> [w941]
            stop <- w961 stop-if-true
            n729 = call <vilib>:"WPI_GyroGetAngle.vi"("GyroDevRef"=w950) -> ("Angle"=w947:dbl)  [unwired: 7 in, 3 out]
            n730 = Bundle("setpoint"=0.0, "Angle"=w947) -> (→"RPM Control Response 4":cluster{"setpoint":dbl, "Angle":dbl})  [unwired: 1 out]
            n731 = Get Date/Time In Seconds() -> (seconds since 1Jan1904=w944:timestamp)
            n732 = Bundle("Prop 4"="Prop 4", "Int 4"="Int 4", "Deriv 4"="Deriv 4") -> (w951:T17)  [unwired: 1 out]
            n733 = To Double Precision Float(number=w944) -> (double precision float=w943:dbl)
            n734 = global read "Robot Global Data.vi" "Avg Wheel Encoder"() -> (w960:dbl)
            n735 = Subtract(x=w943, y=w941) -> (x-y=→"x-y 56":dbl)
            n736 = Bundle("x"=0.7, -0.7) -> (w954:cluster{"x":dbl, dbl})  [unwired: 1 out]
            n737 = call-poly <vilib>:"PID.vi"("output range"=w954, "PID gains"=w951, "process variable"=w947, "setpoint"=0.0) -> ("output"=w945:dbl)  [unwired: 2 in, 5 out]
            "PID Output 4" <- w945
            n738 = Subtract(x=w940, y=w945) -> ()  [unwired: 1 out]
            n739 = Greater Or Equal?(x=w960, y=w959) -> (x >= y?=w961:bool)
            n740 = global write "Robot Global Data.vi" "X Axis Drive Cmd"(w940) -> ()
            n741 = global write "Robot Global Data.vi" "Y Axis Drive Cmd"(w940) -> ()
            n742 = Wait (ms)(milliseconds to wait=u32 10) -> ()  [unwired: 1 out]
          }
        }
        frame #4 {
          # "Stop Drive, Brake,\nand Start up all Conveyors"
          # "Requires State Machine for more than one Ball"
          n743 = disable-structure shown="Disabled" {
            frame Disabled {
              # "Mid Conv Forward"
              # "Lo Conv Forward"
              # "Intake On"
              # "Fire Conv On"
              n744 = global write "Robot Global Data.vi" "Op Button 5"(TRUE ("Op Button 5")) -> ()
              n745 = global write "Robot Global Data.vi" "Op Button 8"(TRUE ("Op Button 5")) -> ()
              n746 = global write "Robot Global Data.vi" "Op Button 2"(TRUE ("Op Button 5")) -> ()
              n747 = global write "Robot Global Data.vi" "Op Button 1"(TRUE ("Op Button 5")) -> ()
            }
            frame Enabled {
            }
          }
          n748 = global write "Robot Global Data.vi" "X Axis Drive Cmd"(w962) -> ()
          n749 = global write "Robot Global Data.vi" "Y Axis Drive Cmd"(w962) -> ()
        }
        frame #5 {
          # "Wait for Ball to reach Prime"
          # "Look for Target"
          n750 = Get Date/Time In Seconds() -> (seconds since 1Jan1904=w967:timestamp)
          n751 = To Double Precision Float(number=w967) -> (double precision float=w968:dbl)
          n752 = while {
            tunnel: w968 -> [w981]
            i -> [w980]
            stop <- w970 stop-if-true
            w975 = 1.0 ("upper limit")
            n753 = global read "Robot Global Data.vi" "Target Angle"() -> (w977:dbl)
            n754 = feedback #31(0) -> (w985:i32)
            "State 3" <- w985
            n755 = feedback #32() -> (w982:dbl)  [unwired: 1 in]
            n756 = case shown="0, Default" w985 {
              tunnel: [w998 w1009 w1016 w1023] -> w978
              tunnel: [0.0 0.5 -0.5 0.5] -> w984
              tunnel: [w995 w1011 0.0 ("Turret Yaw") 0.0 ("Turret Yaw")] -> w983
              tunnel: w982 -> [_ w1011 _ _]
              tunnel: w981 -> [w990 _ _ _]
              frame 0, Default {
                # "Engage Auto-Target\n(take turret to last known target bearing)"
                n757 = Add(x=w990, y=1.0) -> (x+y=w987:dbl)
                n758 = global read "Robot Global Data.vi" "Turret Stable?"() -> (w993:bool)
                "Turret Stable? 3" <- w993
                n759 = Get Date/Time In Seconds() -> (seconds since 1Jan1904=w992:timestamp)
                n760 = global write "Robot Global Data.vi" "Op Button 7"(TRUE ("Op Button 7")) -> ()
                n761 = To Double Precision Float(number=w992) -> (double precision float=w988:dbl)
                n762 = Greater Or Equal?(x=w988, y=w987) -> (x >= y?=w991:bool)
                n763 = Or(x=w991, y=w993) -> (x .or. y?=w994:bool)
                n764 = global read "Robot Global Data.vi" "Turret Yaw"() -> (w995:dbl)
                n765 = Select(t=1, s=w994, f=0) -> (s? t:f=w998:i32)
              }
              frame 1 {
                # "Seek CCW a bit"
                n766 = global read "Robot Global Data.vi" "Left_Limit"() -> (w1001:bool)
                n767 = Subtract(x=w1011, y=15.0) -> (x-y=w1005:dbl)
                n768 = global read "Robot Global Data.vi" "Turret Yaw"() -> (w1006:dbl)
                n769 = Less Or Equal?(x=w1006, y=w1005) -> (x <= y?=w1003:bool)
                n770 = Or(x=w1003, y=w1001) -> (x .or. y?=w1002:bool)
                n771 = global write "Robot Global Data.vi" "Op Button 7"(FALSE ("Op Button 7")) -> ()
                n772 = Select(t=2, s=w1002, f=1) -> (s? t:f=w1009:i32)
              }
              frame 2 {
                # "Search CW"
                n773 = global read "Robot Global Data.vi" "Right_Limit"() -> (w1013:bool)
                n774 = Select(t=3, s=w1013, f=2) -> (s? t:f=w1016:i32)
              }
              frame 3 {
                # "Search CCW"
                n775 = global read "Robot Global Data.vi" "Left_Limit"() -> (w1019:bool)
                n776 = Select(t=2, s=w1019, f=3) -> (s? t:f=w1023:i32)
              }
            }
            n777 = global write "Robot Global Data.vi" "Turret Yaw Joystick Command"(w984) -> ()
            n778 = feedback-in #31(w978) -> ()
            n779 = feedback-in #32(w983) -> ()
            n780 = Negate(x=w975) -> (-x=w976:dbl)
            n781 = In Range and Coerce(upper limit=w975, x=w977, lower limit=w976) -> (In Range?=w974:bool)  [unwired: 1 out]
            "In Range? 3" <- w974
            n782 = global read "Robot Global Data.vi" "Valid Target ?"() -> (w969:bool)
            n783 = global read "Robot Global Data.vi" "PRIME"() -> (w971:bool)
            n784 = call "Stable.vi"("Pulse Width (sec)"="Pulse Width (sec) 3", "Signal Input"=w974) -> ("Stable"=w972:bool)  [unwired: 9 in]
            n785 = Compound Arithmetic op=AND(w972, w971, w969) -> (w970:bool)
            n786 = Wait (ms)(milliseconds to wait=u32 10) -> ()  [unwired: 1 out]
            "Numeric 3" <- w980
          }
        }
        frame #6 {
          # "Stabilize Distance Measurement"
          n787 = Get Date/Time In Seconds() -> (seconds since 1Jan1904=w1026:timestamp)
          n788 = To Double Precision Float(number=w1026) -> (double precision float=w1025:dbl)
          n789 = while {
            tunnel: w1025 -> [w1033]
            stop <- w1036 stop-if-true
            n790 = global read "Robot Global Data.vi" "Target Distance"() -> (w1038:dbl)
            n791 = Get Date/Time In Seconds() -> (seconds since 1Jan1904=w1035:timestamp)
            n792 = To Double Precision Float(number=w1035) -> (double precision float=w1032:dbl)
            n793 = Add(x=w1033, y=4.0) -> (x+y=w1031:dbl)
            n794 = Greater Or Equal?(x=w1032, y=w1031) -> (x >= y?=w1029:bool)
            n795 = feedback #33() -> (w1043:dbl)  [unwired: 1 in]
            n796 = feedback-in #33(w1038) -> ()
            n797 = feedback #34() -> (w1044:dbl)  [unwired: 1 in]
            n798 = feedback-in #34(w1043) -> ()
            n799 = feedback #35() -> (w1045:dbl)  [unwired: 1 in]
            n800 = feedback-in #35(w1044) -> ()
            n801 = feedback #36() -> (w1046:dbl)  [unwired: 1 in]
            n802 = feedback-in #36(w1045) -> ()
            n803 = Bundle("Target Distance"=w1046, "Target Distance"=w1045, "Target Distance"=w1044, "Target Distance"=w1043, "Target Distance"=w1038) -> (w1042:T15)  [unwired: 1 in]
            n804 = Cluster To Array(cluster=w1042) -> (array=w1041:dbl[])
            n805 = call <vilib>:"Std Deviation and Variance.vi"("X"=w1041) -> ("standard deviation"=w1037:dbl)  [unwired: 1 in, 2 out]
            n806 = Less Or Equal?(x=w1037, y=0.3) -> (x <= y?=w1030:bool)
            n807 = Wait (ms)(milliseconds to wait=u32 5) -> ()  [unwired: 1 out]
            n808 = Or(x=w1030, y=w1029) -> (x .or. y?=w1036:bool)
          }
          n809 = global write "Robot Global Data.vi" "Turret Yaw Joystick Command"(0.0 ("Turret Yaw Joystick Command")) -> ()
          n810 = global write "Robot Global Data.vi" "Auto Target"(FALSE ("Auto Target")) -> ()
        }
        frame #7 {
          # "Compute Shooter RPM and set Control value"
          n811 = global read "Robot Global Data.vi" "Target Distance"() -> (w1048:dbl)
          "Target Distance 2" <- w1048
          n812 = global read "Robot Global Data.vi" "Personality"() -> (w1047:string)
          n813 = call "Distance to RPM_V1.vi"("Personality"=w1047, "Target Distance"=w1048) -> ("Shooter RPM Control"=w1049:dbl)  [unwired: 3 in]
          "RPM Control 2" <- w1049
          n814 = global write "Robot Global Data.vi" "Shooter RPM Control"(w1049) -> ()
        }
        frame #8 {
          # "Fire Conv Off"
          n815 = while {
            tunnel: w1051 -> [w1067]
            tunnel: w1050 -> [w1062]
            i -> [w1061]
            stop <- w1066 stop-if-true
            n816 = global read "Robot Global Data.vi" "Shooter Stable?"() -> (w1056:bool)
            n817 = global read "Robot Global Data.vi" "Target Angle"() -> (w1065:dbl)
            n818 = Greater Or Equal?(x=w1061, y=25) -> (x >= y?=w1059:bool)
            n819 = And(x=w1056, y=w1059) -> (x .and. y?=w1054:bool)
            n820 = feedback-in #37(w1056) -> ()
            n821 = feedback #37(TRUE ("Shooter Stable?")) -> (w1057:bool)
            n822 = Absolute Value(x=w1065) -> (abs(x)=w1064:dbl)
            n823 = Greater?(x=w1056, y=w1057) -> (0:w1055:bool)
            n824 = Less Or Equal?(x=w1064, y=w1062) -> (x <= y?=w1063:bool)
            n825 = Or(x=w1055, y=w1054) -> (x .or. y?=w1053:bool)
            n826 = Get Date/Time In Seconds() -> (seconds since 1Jan1904=w1070:timestamp)
            n827 = To Double Precision Float(number=w1070) -> (double precision float=w1069:dbl)
            n828 = Subtract(x=w1069, y=w1067) -> (x-y=→"x-y 60":dbl)
            n829 = And(x=w1053, y=w1063) -> (x .and. y?=w1066:bool)
            n830 = Wait (ms)(milliseconds to wait=u32 10) -> ()  [unwired: 1 out]
          }
          n831 = global write "Robot Global Data.vi" "Op Button 5"(FALSE ("Op Button 5")) -> ()
        }
        frame #9 {
          # "Fire"
          # "Fire Ball 1"
          n832 = while {
            tunnel: "Bridge Ball Timeout (sec) 4" -> [w1078]
            tunnel: w1073 -> [w1076]
            stop <- w1079 stop-if-true
            n833 = global read "Robot Global Data.vi" "PRIME"() -> (w1082:bool)
            n834 = Wait (ms)(milliseconds to wait=u32 10) -> ()  [unwired: 1 out]
            n835 = Not(x=w1082) -> (.not. x?=w1081:bool)
            n836 = Get Date/Time In Seconds() -> (seconds since 1Jan1904=w1084:timestamp)
            n837 = Add(x=w1076, y=w1078) -> (x+y=w1083:dbl)
            n838 = To Double Precision Float(number=w1084) -> (double precision float=w1077:dbl)
            n839 = Greater Or Equal?(x=w1077, y=w1083) -> (x >= y?=w1080:bool)
            n840 = Subtract(x=w1077, y=w1076) -> (x-y=→"x-y 61":dbl)
            n841 = Or(x=w1080, y=w1081) -> (x .or. y?=w1079:bool)
          }
          n842 = global write "Robot Global Data.vi" "Op Button 5"(TRUE ("Op Button 5")) -> ()
        }
        frame #10 {
          # "Re prime for Ball 2"
          n843 = disable-structure shown="Disabled" {
            frame Disabled {
              # "Mid Conv Forward"
              # "Fire Conv On"
              n844 = global write "Robot Global Data.vi" "Op Button 5"(TRUE ("Op Button 5")) -> ()
              n845 = global write "Robot Global Data.vi" "Op Button 1"(TRUE ("Op Button 5")) -> ()
            }
            frame Enabled {
            }
          }
          n846 = while {
            stop <- w1089 stop-if-true
            n847 = global read "Robot Global Data.vi" "PRIME"() -> (w1089:bool)
            n848 = Wait (ms)(milliseconds to wait=u32 10) -> ()  [unwired: 1 out]
          }
          n849 = global write "Robot Global Data.vi" "Op Button 5"(FALSE ("Op Button 5")) -> ()
        }
        frame #11 {
          # "May need to test for Ready & Stable,\notherwise may fire on control overshoot"
          # "Wait for Shooter to reach RPM"
          n850 = while {
            tunnel: w1093 -> [w1109]
            tunnel: "Ball 1 Timeout (sec) 5" -> [w1110]
            tunnel: w1091 -> [w1105]
            i -> [w1104]
            stop <- w1114 stop-if-true
            # "Timeout"
            # "Do Nothing 'til Shooter is at speed"
            n851 = global read "Robot Global Data.vi" "Shooter Stable?"() -> (w1099:bool)
            n852 = global read "Robot Global Data.vi" "Target Angle"() -> (w1107:dbl)
            n853 = Greater Or Equal?(x=w1104, y=25) -> (x >= y?=w1102:bool)
            n854 = Get Date/Time In Seconds() -> (seconds since 1Jan1904=w1115:timestamp)
            n855 = And(x=w1099, y=w1102) -> (x .and. y?=w1097:bool)
            n856 = feedback-in #38(w1099) -> ()
            n857 = feedback #38(TRUE ("Shooter Stable?")) -> (w1100:bool)
            n858 = To Double Precision Float(number=w1115) -> (double precision float=w1116:dbl)
            n859 = Greater?(x=w1099, y=w1100) -> (0:w1098:bool)
            n860 = Absolute Value(x=w1107) -> (abs(x)=w1108:dbl)
            n861 = Subtract(x=w1116, y=w1109) -> (x-y=→"x-y 42":dbl)
            n862 = Or(x=w1098, y=w1097) -> (x .or. y?=w1096:bool)
            n863 = Less Or Equal?(x=w1108, y=w1105) -> (x <= y?=w1106:bool)
            n864 = And(x=w1096, y=w1106) -> (x .and. y?=w1095:bool)
            n865 = Get Date/Time In Seconds() -> (seconds since 1Jan1904=w1112:timestamp)
            n866 = Wait (ms)(milliseconds to wait=u32 10) -> ()  [unwired: 1 out]
            n867 = Add(x=w1109, y=w1110) -> (x+y=w1111:dbl)
            n868 = To Double Precision Float(number=w1112) -> (double precision float=w1113:dbl)
            n869 = Greater Or Equal?(x=w1113, y=w1111) -> (x >= y?=w1094:bool)
            n870 = Or(x=w1095, y=w1094) -> (x .or. y?=w1114:bool)
          }
        }
        frame #12 {
          # "Bridge Down"
          n871 = global write "Robot Global Data.vi" "Dr Button 2"(FALSE ("Dr Button 5")) -> ()
          n872 = global write "Robot Global Data.vi" "X Axis Drive Cmd"(w1120) -> ()
          n873 = global write "Robot Global Data.vi" "Y Axis Drive Cmd"(w1120) -> ()
        }
        frame #13 {
          # "Ensure Fire 'Button' has gone\nFalse (Pulse Stretcher complete)\nbefore attempting to Fire again."
          n874 = while {
            stop <- w1122 continue-if-true
            n875 = global read "Robot Global Data.vi" "Report Fire"() -> (w1122:bool)
            n876 = Wait (ms)(milliseconds to wait=u32 10) -> ()  [unwired: 1 out]
          }
        }
        frame #14 {
          # "Fire"
          # "Will PRIME turn off too early, \nbefore ball has left the Shooter?"
          # "Fire Ball 2"
          n877 = while {
            tunnel: w1124 -> [w1127]
            stop <- w1125 continue-if-true
            n878 = Wait (ms)(milliseconds to wait=u32 10) -> ()  [unwired: 1 out]
            n879 = global read "Robot Global Data.vi" "PRIME"() -> (w1125:bool)
            n880 = Get Date/Time In Seconds() -> (seconds since 1Jan1904=w1129:timestamp)
            n881 = To Double Precision Float(number=w1129) -> (double precision float=w1128:dbl)
            n882 = Subtract(x=w1128, y=w1127) -> (x-y=→"x-y 43":dbl)
          }
          n883 = global write "Robot Global Data.vi" "Op Button 5"(TRUE ("Op Button 5")) -> ()
        }
        frame #15 {
          # "Fire"
          n884 = global write "Robot Global Data.vi" "Collector State Machine"(TRUE ("Collector State Machine")) -> ()
          n885 = global write "Robot Global Data.vi" "Op Button 5"(FALSE ("Op Button 5")) -> ()
        }
        frame #16 {
          # "Ensure Fire 'Button' has gone\nFalse (Pulse Stretcher complete)\nbefore attempting to Fire again."
          n886 = while {
            stop <- w1134 continue-if-true
            n887 = global read "Robot Global Data.vi" "Report Fire"() -> (w1134:bool)
            n888 = Wait (ms)(milliseconds to wait=u32 10) -> ()  [unwired: 1 out]
          }
        }
        frame #17 {
          n889 = while {
            tunnel: w1135 -> [w1136]
            stop <- FALSE stop-if-true
            # "Fire"
            n890 = global read "Robot Global Data.vi" "Shooter Stable?"() -> (w1139:bool)
            n891 = global read "Robot Global Data.vi" "PRIME"() -> (w1140:bool)
            n892 = global read "Robot Global Data.vi" "Target Angle"() -> (w1142:dbl)
            n893 = Absolute Value(x=w1142) -> (abs(x)=w1141:dbl)
            n894 = Less Or Equal?(x=w1141, y=w1136) -> (x <= y?=w1138:bool)
            n895 = Compound Arithmetic op=AND(w1140, w1139, w1138) -> (w1137:bool)
            n896 = global write "Robot Global Data.vi" "Op Button 5"(w1137) -> ()
            n897 = Wait (ms)(milliseconds to wait=u32 10) -> ()  [unwired: 1 out]
          }
        }
      }
    }
  }
